vi "A170316-11_Auto.vi"() -> ()   [LabVIEW 2020]
uses:
  2e0b5f5e-2208-4490-a798-25a802626be8.vi
  Global_Variable/A170316-11.vi
  Global_Variable/Global.vi
  Database/Global1.vi
  <vilib>/addons/database/Connection.llb/DB Tools Open Connec (String).vi
  <vilib>/addons/database/NI_Database_API.lvlib
  <vilib>/regexp/Match Regular Expression.xnode
panel:
  out "设备状态":u16
  out "请拾取O型圈":bool
  out "请拾取弹簧":bool
  in  "控制器支架":T1(ring)
  in  "ECU步骤":T2(ring)
  in  "装配步骤":T3(ring)
  out "产品型号":string
  in  "更换产品":refnum<vi>
  in  "前序OK？_ECU":string
  in  "前序OK？":string
  in  "Process":string[](array[string])
  in  "Code":string[](array[string])
  in  "User":string[](array[string])
  in  "Result":string[](array[string])
  in  "Device":string[](array[string])
  out "请安装挡片":bool
  in  "STEP2":string
  in  "STEP1":string
  out "请取降噪块1":bool
  out "电机安装螺栓3扭矩确认":bool
  out "控制器支架螺栓5拧紧确认":bool
  out "安装扎带并取走工件":bool
  out "涂色标":bool
  out "按启动按钮拍照确认":bool
  out "电机安装螺栓2扭矩确认":bool
  out "电机安装螺栓1扭矩确认":bool
  out "请安装锁紧螺母":bool
  out "请取降噪垫片2":bool
  out "请取降噪垫片1":bool
  out "请取锁紧块":bool
  out "安装弹性垫圈弹簧并按启动拍照":bool
  out "请取降噪块2":bool
  out "控制器支架涂色标":bool
  out "控制器支架螺栓4拧紧确认":bool
  out "控制器支架螺栓3拧紧确认":bool
  out "控制器支架螺栓2拧紧确认":bool
  out "控制器支架螺栓1拧紧确认":bool
  out "请安装推力滚针轴承":bool
  in  "更换布局":string
  out "请拍照确认":bool
  out "安装支架扎带安装":bool
  out "请安装弹簧":bool
  out "控制器支架安装线卡扎带":bool
  out "磨合次数":i32
  in  "判定结果":bool[][](array[boolean])=[[TRUE]]
  in  "STEP3":string
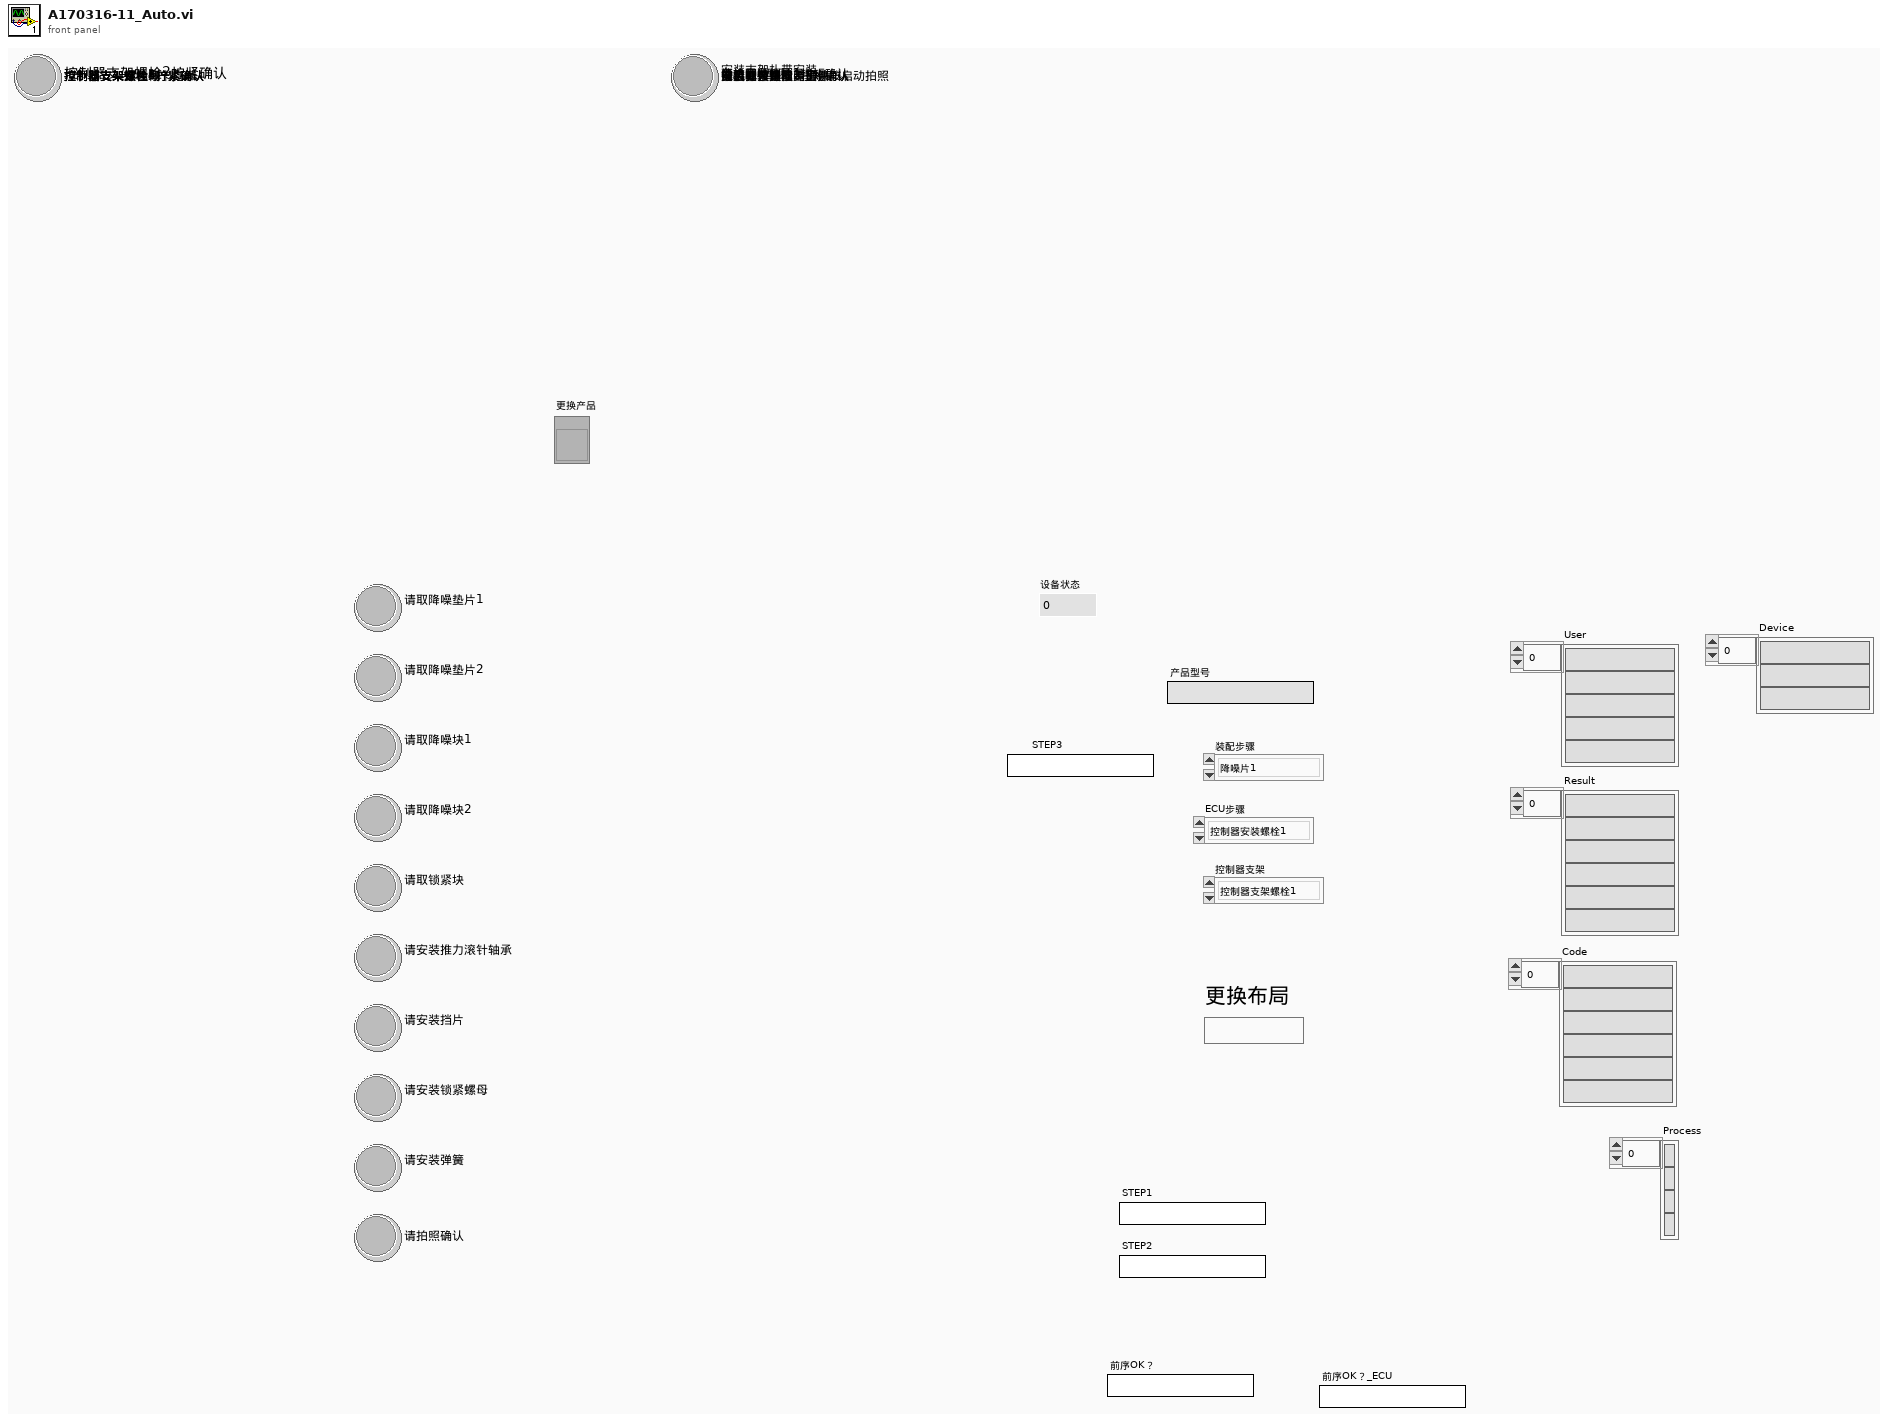
[diagram p1: front panel]
types:
  T1 = enum16{"控制器支架螺栓1", "控制器支架螺栓2", "控制器支架螺栓3", "控制器支架螺栓4", "控制器支架螺栓5", "涂色标", "安装线卡轧带", "完成"}
  T2 = enum16{"控制器安装螺栓1", "控制器安装螺栓2", "控制器安装螺栓3", "安装支架螺栓1", "安装支架螺栓2", "安装支架螺栓3", "安装支架螺栓4", "涂色标", "安装线卡轧带", "取走工件", "完成"}
  T3 = enum16{"降噪片1", "降噪片2", "降噪块1", "降噪块2", "锁紧块", "滚针轴承", "垫片", "锁紧螺母", "弹簧", "轴承拍照", "完成"}
  T4 = cluster{i64, i64, i64, "装配结果":string, "result string":string}
  T5 = cluster{i64, i64, i64, "装配结果":string, "result string":string}[]
  T6 = typedef "NI_Database_API.lvlib/Conn ObjectReference.ctl" = refnum<k1>
  T7 = cluster{i64, i64, i64, "ECU工位生产结果":string, "result string":string}
  T8 = cluster{i64, i64, i64, "ECU工位生产结果":string, "result string":string}[]
  T9 = cluster{"ECU工位生产结果":string, "result string":string}
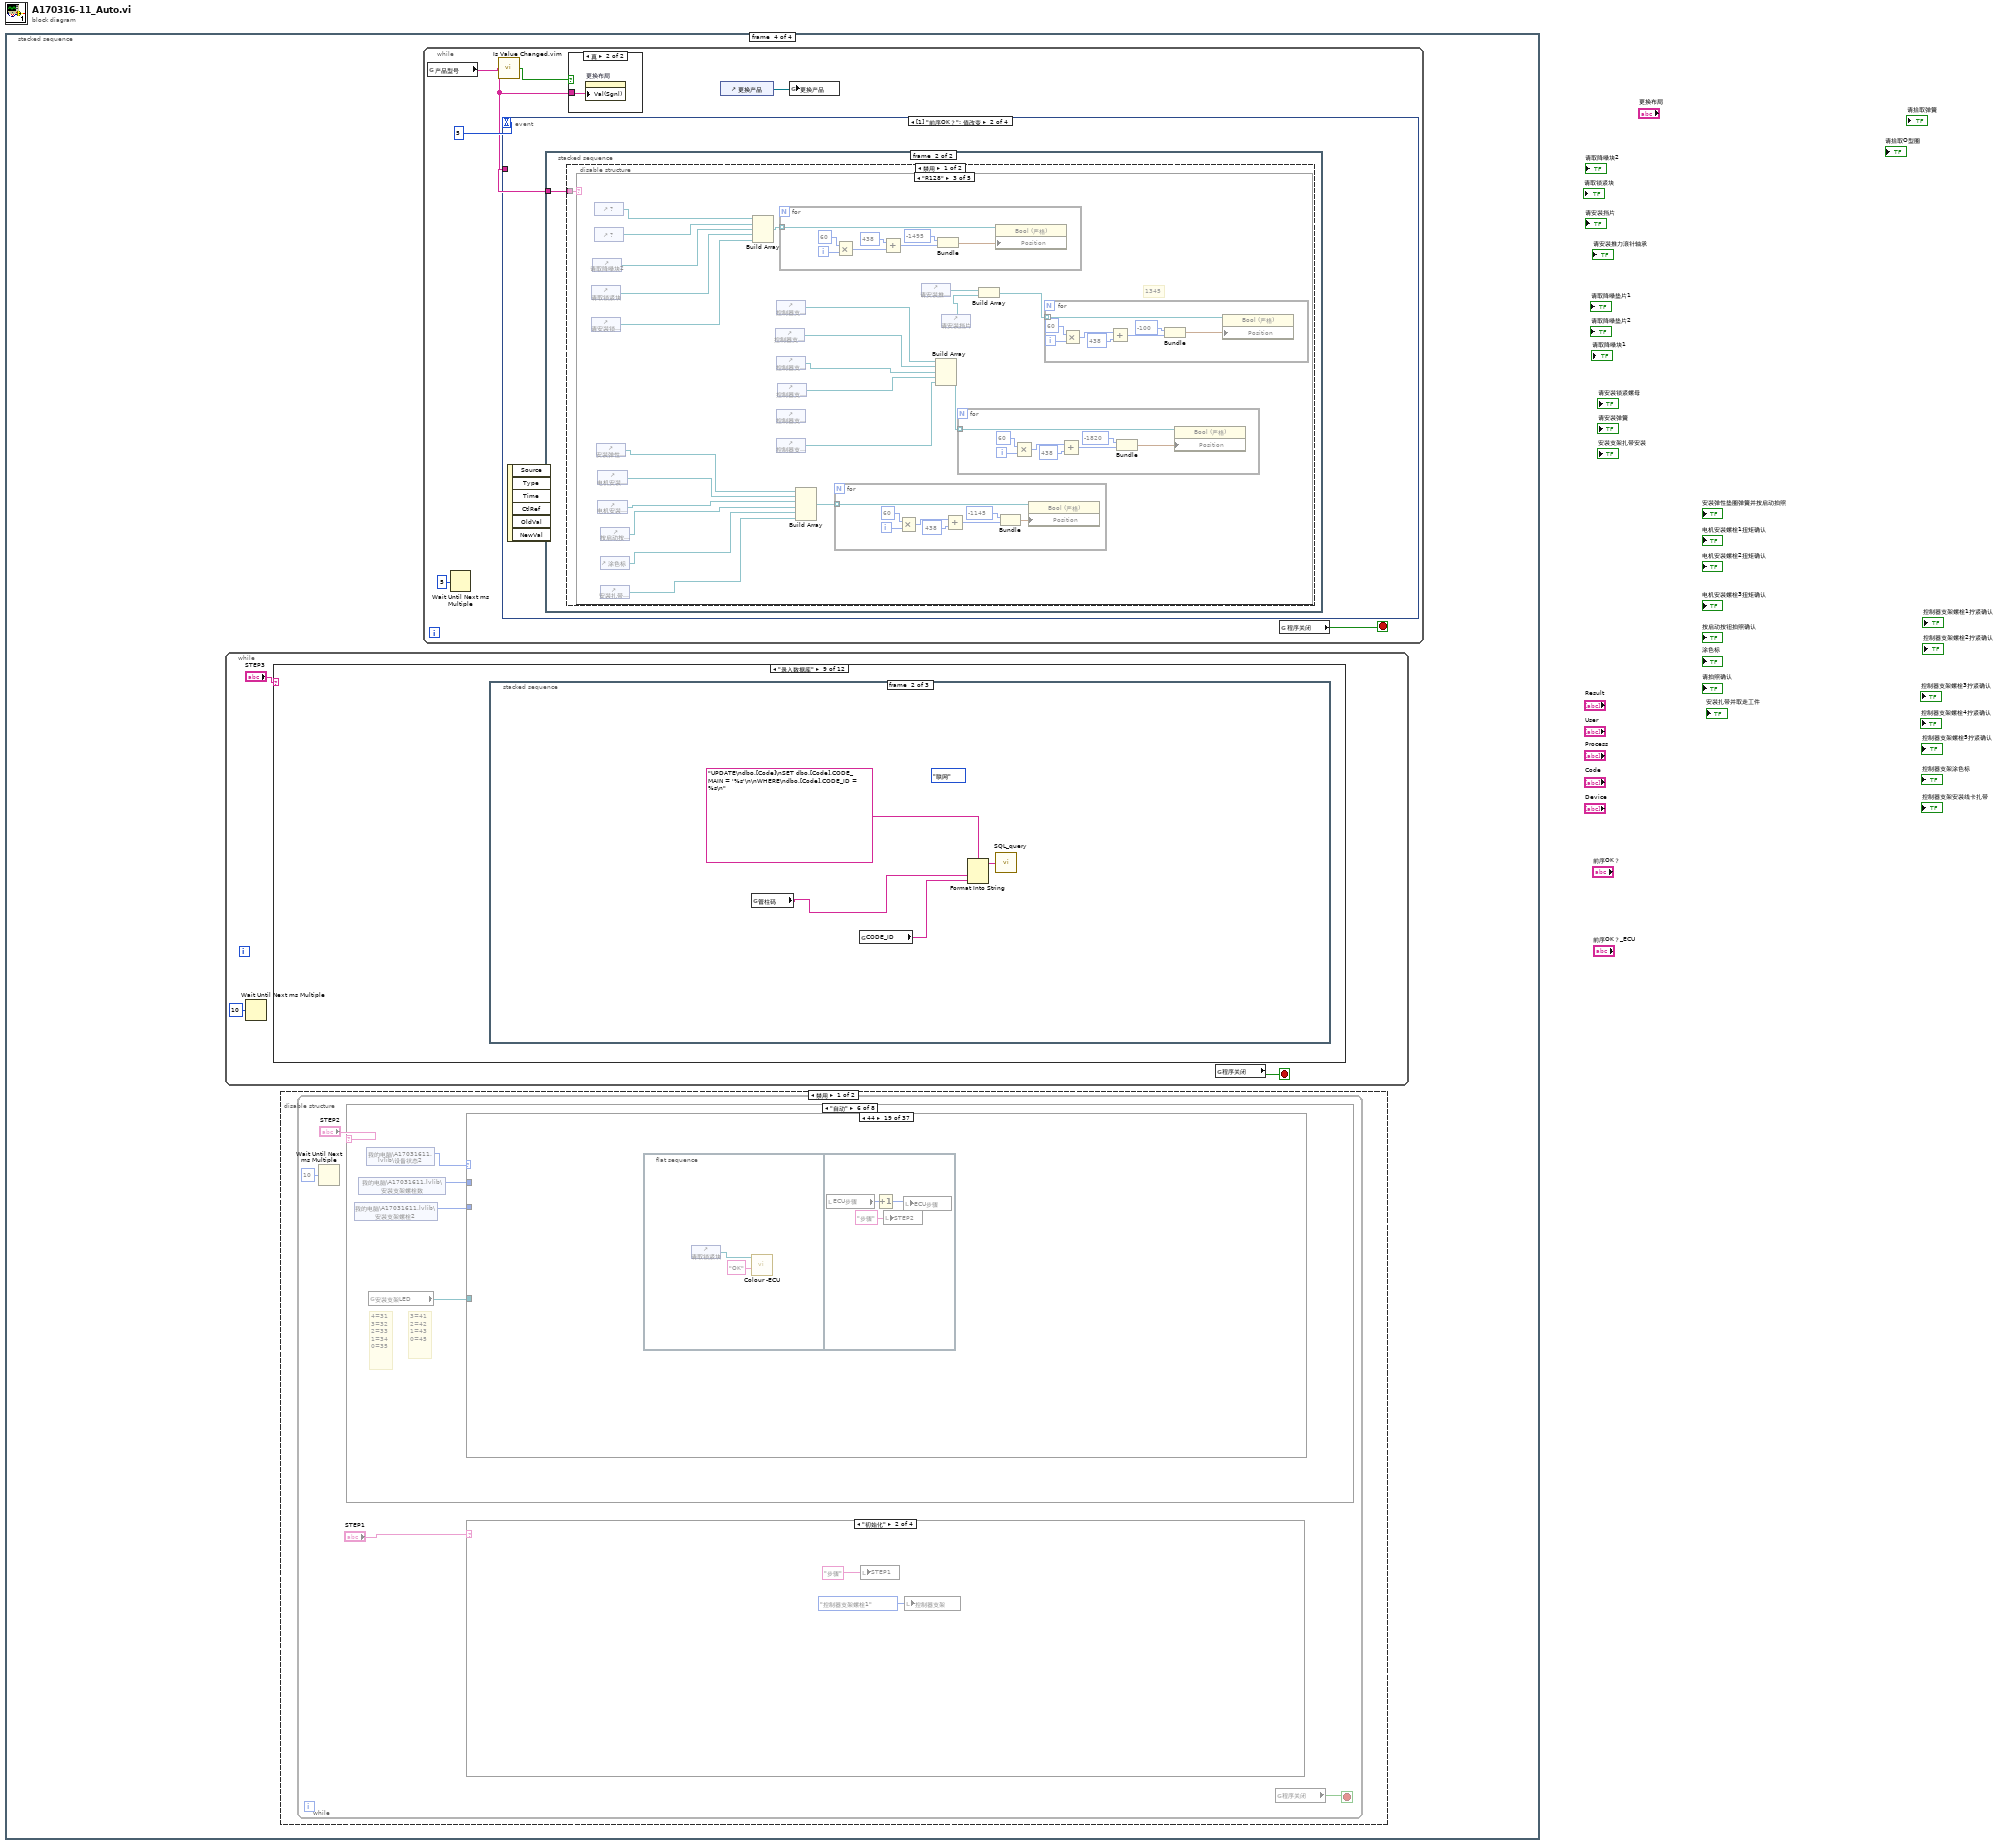
[diagram p0: block diagram]
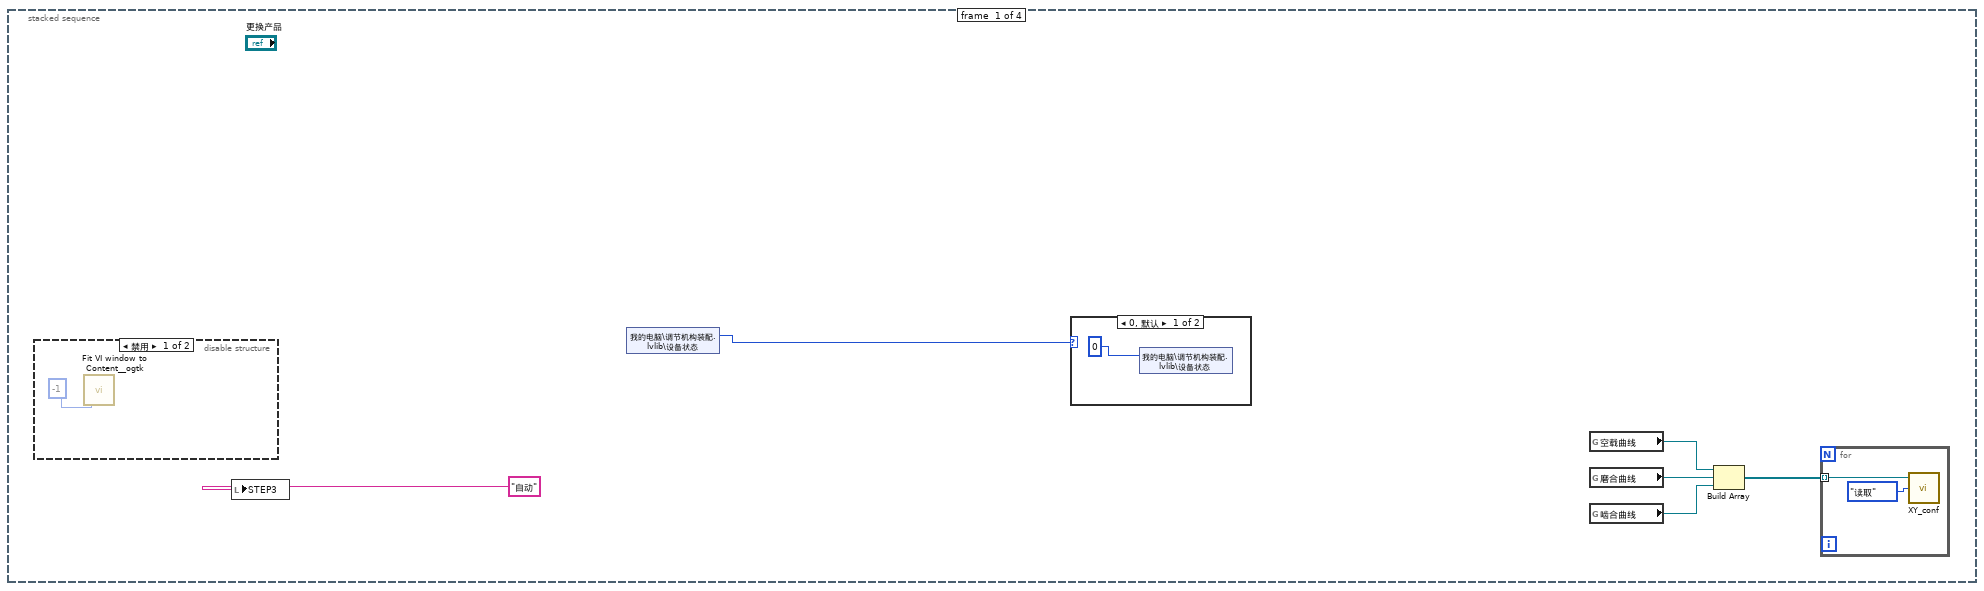
[diagram p2: hidden frame]
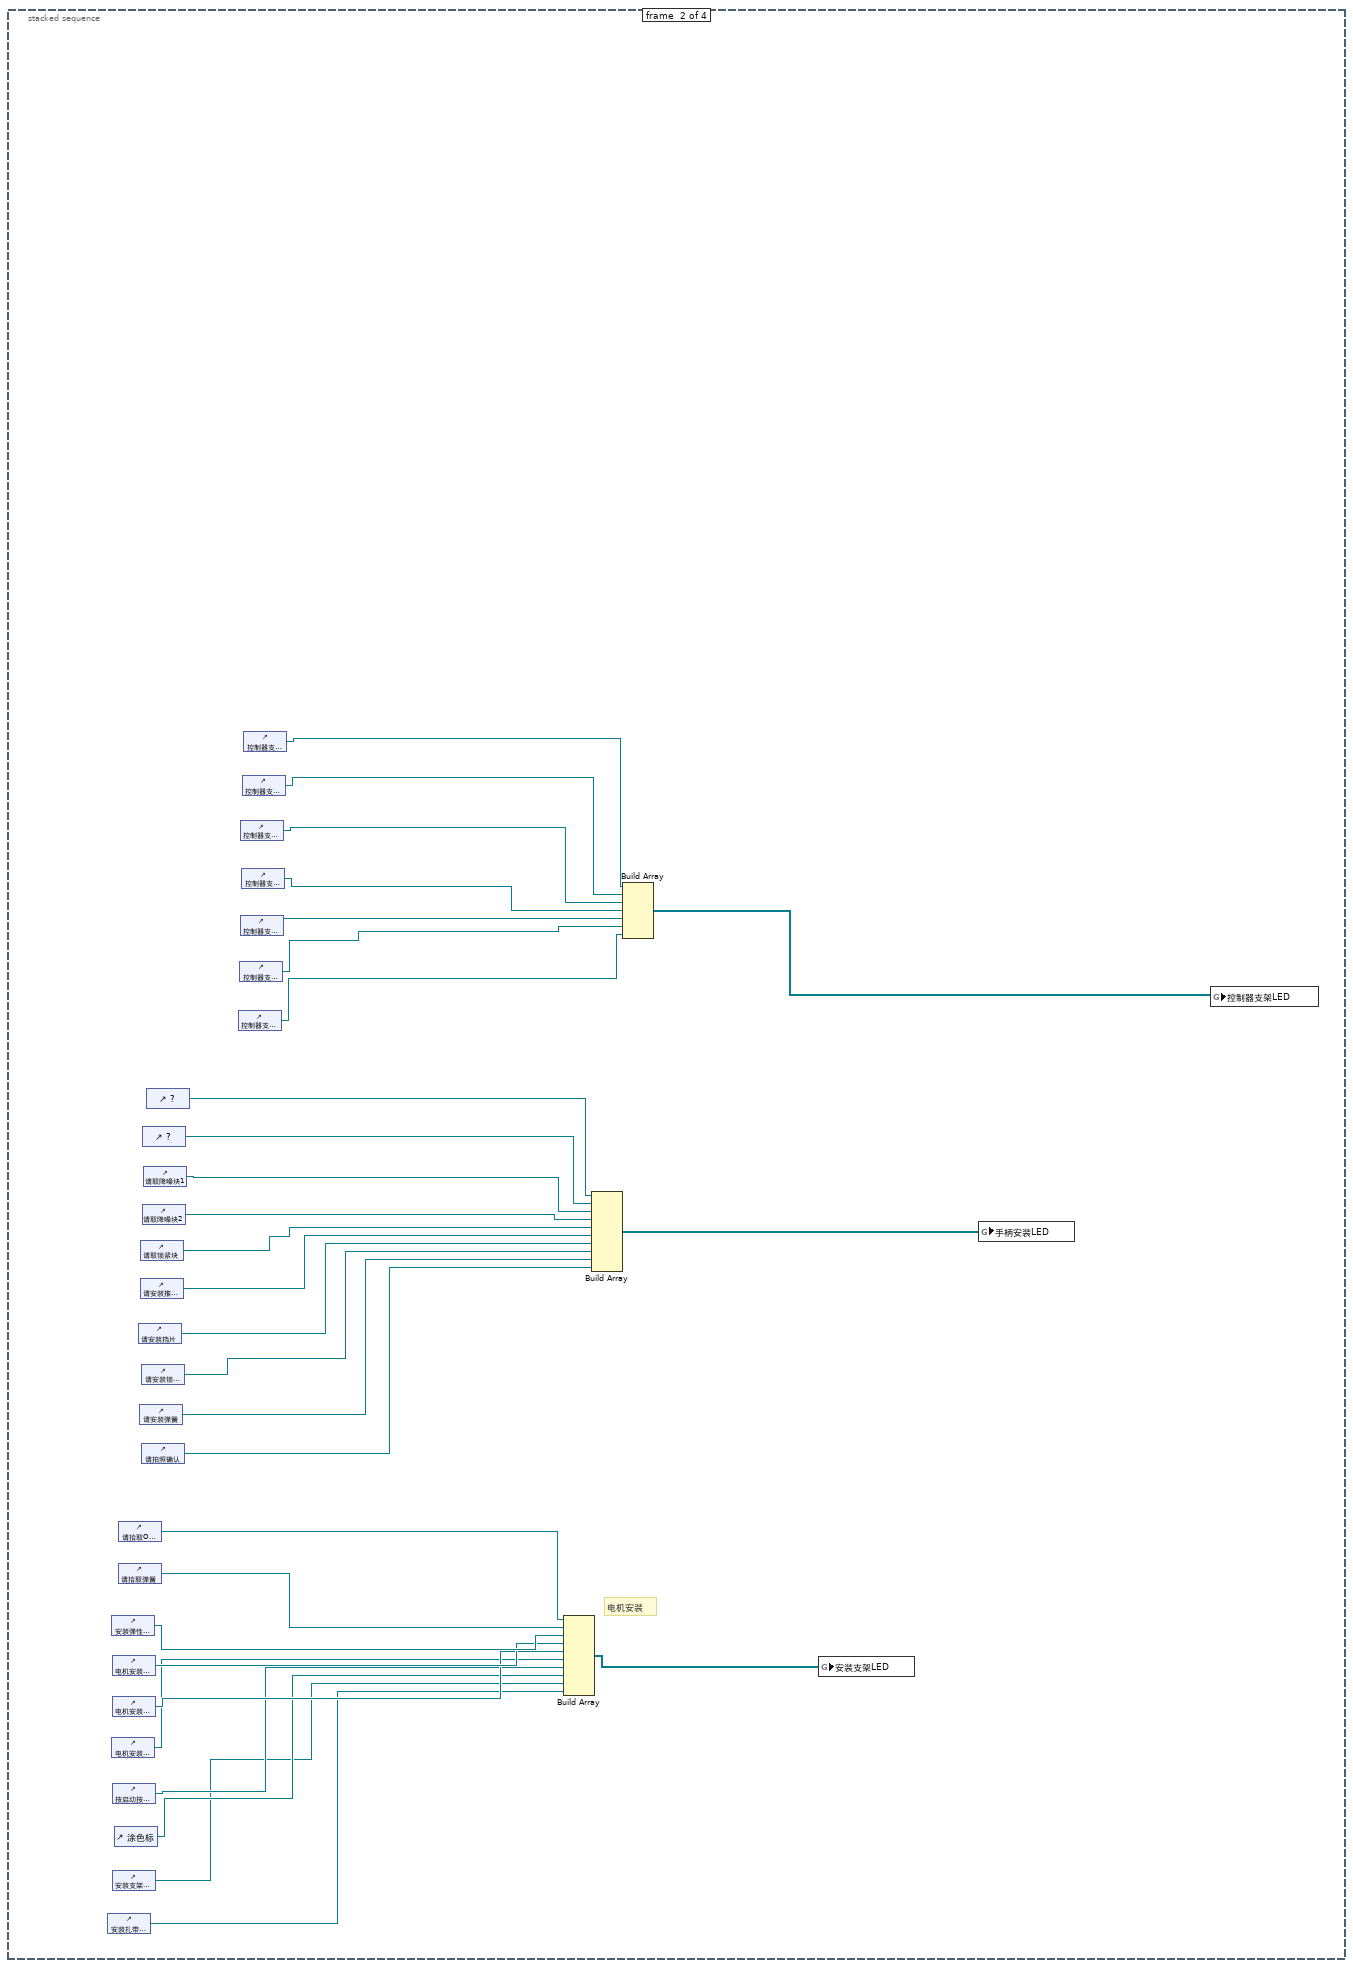
[diagram p5: hidden frame]
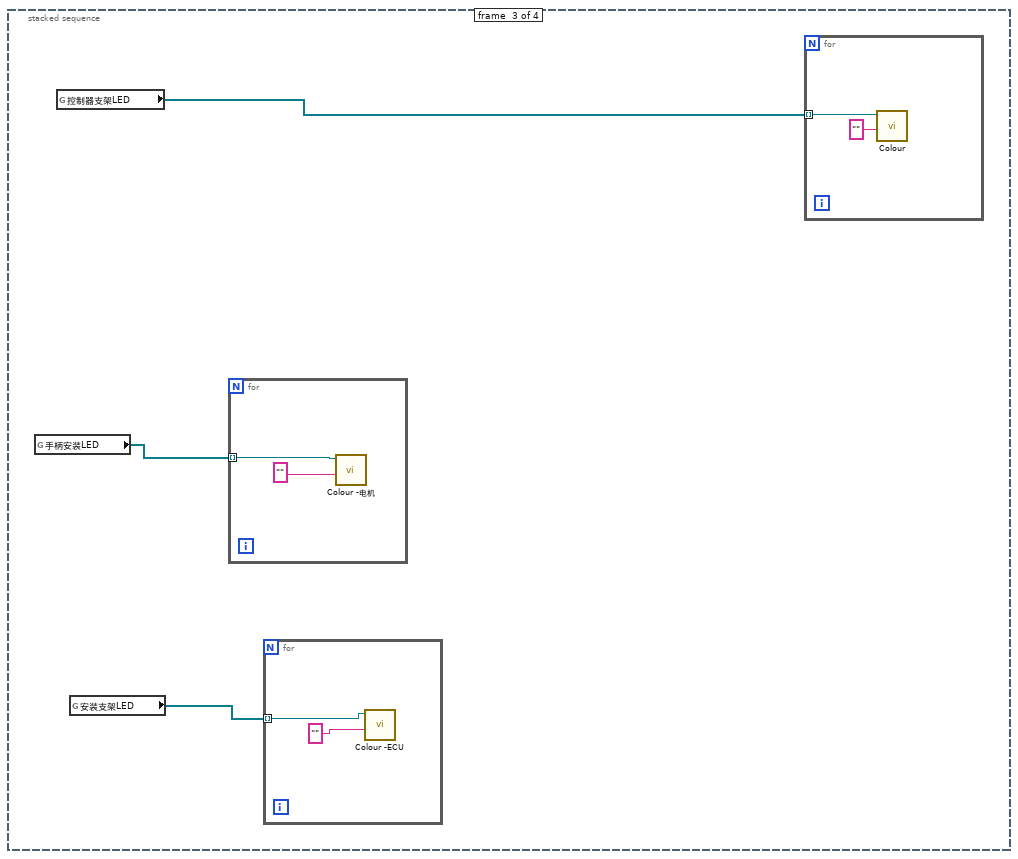
[diagram p6: hidden frame]
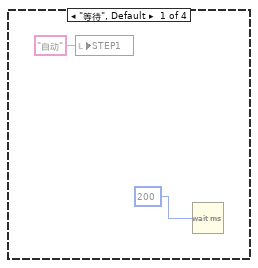
[diagram p7: hidden frame]
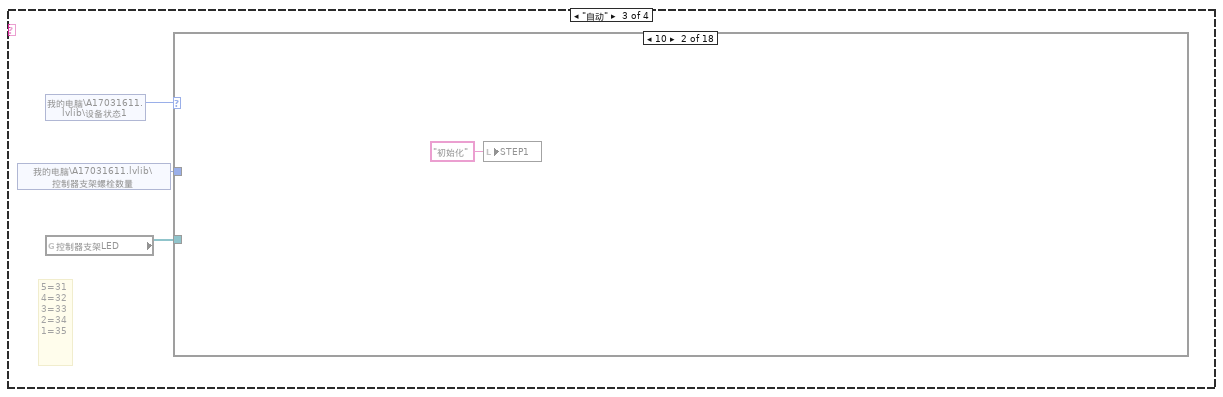
[diagram p8: hidden frame]
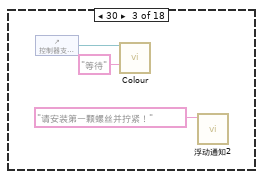
[diagram p10: hidden frame]
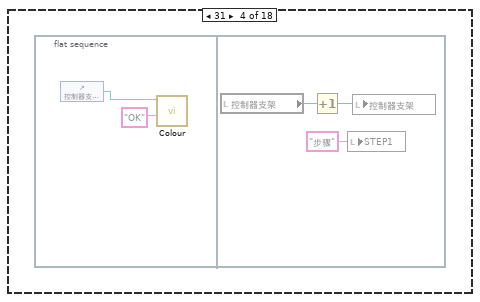
[diagram p11: hidden frame]
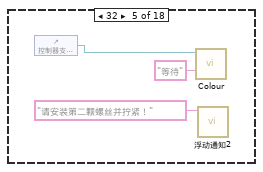
[diagram p12: hidden frame]
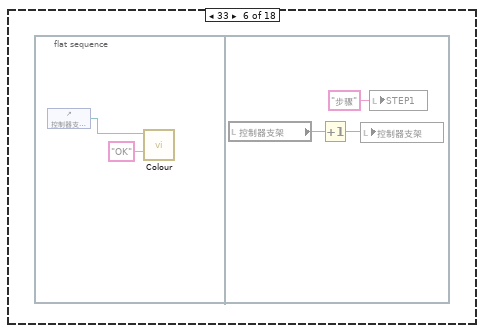
[diagram p13: hidden frame]
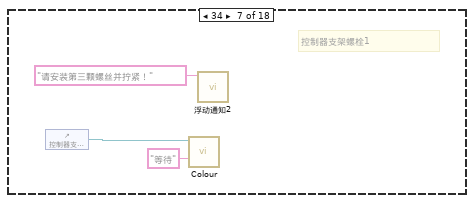
[diagram p14: hidden frame]
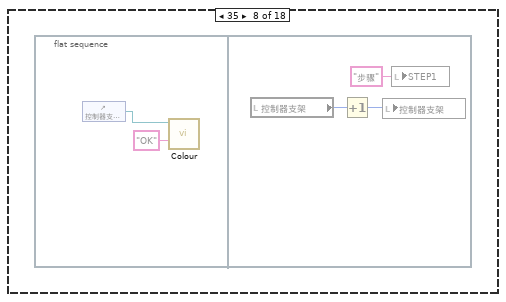
[diagram p15: hidden frame]
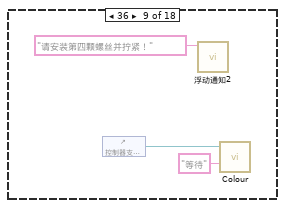
[diagram p16: hidden frame]
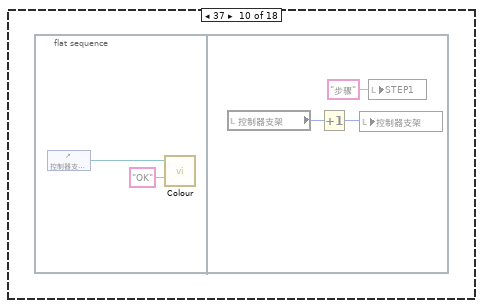
[diagram p17: hidden frame]
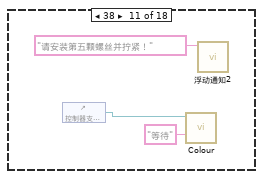
[diagram p18: hidden frame]
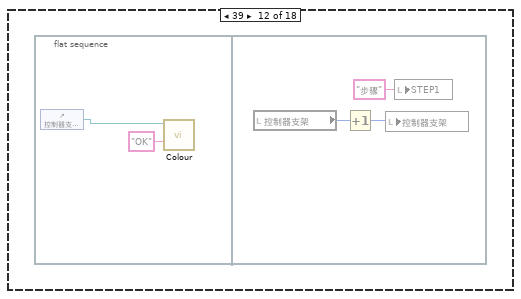
[diagram p19: hidden frame]
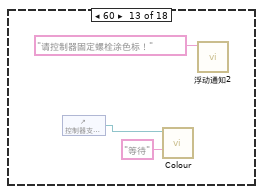
[diagram p20: hidden frame]
diagram:
  n1 = stacked-sequence {
    frame #0 {
      n2 = disable-structure shown="禁用" {
        frame Disabled {
          n3 = call "Fit VI window to Content__ogtk.vi"("border spacing (2 px)"=-1) -> ()  [unwired: 5 in, 2 out]
        }
        frame Enabled {
        }
      }
      n4 = local write "STEP3"("自动" ("STEP")) -> ()
      n5 = shared-variable "我的电脑\\调节机构装配.lvlib\\设备状态"() -> (w1:u16)  [unwired: 1 in, 1 out]
      n6 = case shown="0, 默认" w1 {
        frame 0, Default {
          n7 = shared-variable "我的电脑\\调节机构装配.lvlib\\设备状态"(i16 0 ("设备状态")) -> ()  [unwired: 1 in, 1 out]
        }
        frame 3721..3723 {
        }
      }
      n8 = global read "A170316-11.vi" "空载曲线"() -> (w2:refnum<vi>)
      n9 = global read "A170316-11.vi" "磨合曲线"() -> (w3:refnum<vi>)
      n10 = global read "A170316-11.vi" "啮合曲线"() -> (w4:refnum<vi>)
      n11 = Build Array(w2, w3, w4) -> (w5:refnum<vi>[])
      n12 = for {
        tunnel: w5 -> [w10] mode=indexing
        n13 = call "XY_conf.vi"("方式"=enum16{"写入", "读取"}."读取", "XY图引用"=w10) -> ()  [unwired: 3 in, 1 out]
      }
    }
    frame #1 {
      # "电机安装"
      n14 = control-ref of="安装扎带并取走工件"() -> (w25:refnum<vi>)
      n15 = control-ref of="安装弹性垫圈弹簧并按启动拍照"() -> (w32:refnum<vi>)
      n16 = control-ref of="电机安装螺栓3扭矩确认"() -> (w29:refnum<vi>)
      n17 = control-ref of="电机安装螺栓1扭矩确认"() -> (w31:refnum<vi>)
      n18 = control-ref of="电机安装螺栓2扭矩确认"() -> (w30:refnum<vi>)
      n19 = control-ref of="按启动按钮拍照确认"() -> (w28:refnum<vi>)
      n20 = control-ref of="安装支架扎带安装"() -> (w26:refnum<vi>)
      n21 = control-ref of="涂色标"() -> (w27:refnum<vi>)
      n22 = control-ref of="请拾取O型圈"() -> (w13:refnum<vi>)
      n23 = control-ref of="请拾取弹簧"() -> (w14:refnum<vi>)
      n24 = control-ref of="请安装挡片"() -> (w18:refnum<vi>)
      n25 = control-ref of="请安装弹簧"() -> (w16:refnum<vi>)
      n26 = control-ref of="请取锁紧块"() -> (w20:refnum<vi>)
      n27 = control-ref of="请安装推力滚针轴承"() -> (w19:refnum<vi>)
      n28 = control-ref of="请安装锁紧螺母"() -> (w17:refnum<vi>)
      n29 = control-ref of="请拍照确认"() -> (w15:refnum<vi>)
      n30 = control-ref of="?"() -> (w23:refnum<vi>)
      n31 = control-ref of="请取降噪块2"() -> (w21:refnum<vi>)
      n32 = control-ref of="请取降噪块1"() -> (w22:refnum<vi>)
      n33 = control-ref of="?"() -> (w24:refnum<vi>)
      n34 = control-ref of="控制器支架安装线卡扎带"() -> (w33:refnum<vi>)
      n35 = control-ref of="控制器支架涂色标"() -> (w34:refnum<vi>)
      n36 = control-ref of="控制器支架螺栓3拧紧确认"() -> (w37:refnum<vi>)
      n37 = control-ref of="控制器支架螺栓5拧紧确认"() -> (w35:refnum<vi>)
      n38 = control-ref of="控制器支架螺栓4拧紧确认"() -> (w36:refnum<vi>)
      n39 = control-ref of="控制器支架螺栓2拧紧确认"() -> (w38:refnum<vi>)
      n40 = control-ref of="控制器支架螺栓1拧紧确认"() -> (w39:refnum<vi>)
      n41 = Build Array(w13, w14, w32, w31, w30, w29, w28, w27, w26, w25) -> (w11:refnum<vi>[])
      n42 = Build Array(w24, w23, w22, w21, w20, w19, w18, w17, w16, w15) -> (w12:refnum<vi>[])
      n43 = Build Array(w39, w38, w37, w36, w35, w34, w33) -> (w40:refnum<vi>[])
      n44 = global write "A170316-11.vi" "安装支架LED"(w11) -> ()
      n45 = global write "A170316-11.vi" "手柄安装LED"(w12) -> ()
      n46 = global write "A170316-11.vi" "控制器支架LED"(w40) -> ()
    }
    frame #2 {
      n47 = global read "A170316-11.vi" "手柄安装LED"() -> (w42:refnum<vi>[])
      n48 = global read "A170316-11.vi" "控制器支架LED"() -> (w43:refnum<vi>[])
      n49 = global read "A170316-11.vi" "安装支架LED"() -> (w41:refnum<vi>[])
      n50 = for {
        tunnel: w42 -> [w47] mode=indexing
        n51 = call "Colour -电机.vi"("result"="", "colourRef"=w47) -> ()  [unwired: 9 in, 1 out]
      }
      n52 = for {
        tunnel: w41 -> [w45] mode=indexing
        n53 = call "Colour -ECU.vi"("result"="", "colourRef"=w45) -> ()  [unwired: 9 in, 1 out]
      }
      n54 = for {
        tunnel: w43 -> [w48] mode=indexing
        n55 = call "Colour.vi"("result"="", "colourRef"=w48) -> ()  [unwired: 9 in, 1 out]
      }
    }
    frame #3 {
      n56 = while {
        stop <- w633 stop-if-true
        n57 = Wait Until Next ms Multiple(millisecond multiple=u32 10 ("毫秒倍数")) -> ()  [unwired: 1 out]
        n58 = case shown="\"录入数据库\"" "STEP3" {
          frame "等待", Default {
            n59 = local write "STEP3"("自动" ("STEP")) -> ()
            n60 = Wait (ms)(milliseconds to wait=u32 200 ("等待时间（毫秒）")) -> ()  [unwired: 1 out]
          }
          frame "手动" {
            n61 = global read "Global.vi" "ECU自动"() -> (w640:refnum<vi>)
            n62 = property class="Bool (严格)"(reference=w640, "Value"=FALSE) -> ()  [unwired: 1 in, 2 out]
            n63 = local write "STEP1"("等待" ("STEP1")) -> ()
            n64 = shared-variable "我的电脑\\调节机构装配.lvlib\\设备状态"(u16 0 ("设备状态")) -> ()  [unwired: 1 in, 1 out]
            n65 = global read "Global.vi" "电机程序自动"() -> (w642:refnum<vi>)
            n66 = property class="Bool"(reference=w642, "Value"=FALSE) -> ()  [unwired: 1 in, 2 out]
            n67 = local write "STEP3"("等待" ("STEP")) -> ()
            n68 = Wait (ms)(milliseconds to wait=u32 100 ("等待时间（毫秒）")) -> ()  [unwired: 1 out]
          }
          frame "初始化" {
            n69 = stacked-sequence {
              frame #0 {
                w655 = enum16{"录入", "清空"}."清空" ("功能")
                n70 = global read "Global.vi" "装配前序显示字"() -> (w646:refnum<vi>)
                n71 = shared-variable "我的电脑\\Global.lvlib\\工位追溯码"("" ("传感器码")) -> ()  [unwired: 1 in, 1 out]
                n72 = call "物料信息录入.vi"("功能"=w655) -> ("错误输出"=w654:errorcluster)  [unwired: 14 in]
                n73 = call "质量信息录入.vi"("功能"=w655, "错误输入（无错误）"=w654) -> ("错误输出"=w656:errorcluster)  [unwired: 13 in]
                n74 = property class="Str"(reference=w646, "Value"="" ("值")) -> (reference out=w645:refnum<vi>)  [unwired: 1 in, 1 out]
                n75 = call "不合格信息录入.vi"("功能"=w655, "错误输入（无错误）"=w656) -> ()  [unwired: 13 in, 1 out]
                n76 = property class="Str"(reference=w645, "Text.BGColor"=u32 16777216 ("文本.文本颜色:背景色")) -> ()  [unwired: 1 in, 2 out]
                n77 = global read "Global.vi" "电机程序自动"() -> (w652:refnum<vi>)
                n78 = global read "Global.vi" "检测结果"() -> (w650:refnum<vi>)
                n79 = property class="Bool"(reference=w652, "Value"=TRUE) -> ()  [unwired: 1 in, 2 out]
                n80 = call "Colour.vi"("result"="", "colourRef"=w650) -> ()  [unwired: 9 in, 1 out]
              }
              frame #1 {
                n81 = global read "A170316-11.vi" "手柄安装LED"() -> (w657:refnum<vi>[])
                n82 = for {
                  tunnel: w657 -> [w659] mode=indexing
                  n83 = call "Colour -电机.vi"("result"="", "colourRef"=w659) -> ()  [unwired: 9 in, 1 out]
                }
              }
              frame #2 {
                n84 = global read "Global.vi" "Result"() -> (w663:refnum<vi>)
                n85 = property class="Tbl"(reference=w663, "Value"=string[][] []) -> (reference out=w664:refnum<vi>, error out=w665:errorcluster)  [unwired: 1 in]
                n86 = property class="Tbl"(reference=w664, error in=w665, "Row Headers[]"=string[] ["正向空载扭矩最大值", "正向空载扭矩最小值", "正向空载扭矩平均值", "正向空载扭矩波动值", "逆向空载扭矩最大值", "逆向空载扭矩最小值", "逆向空载扭矩平均值", "逆向空载扭矩波动值", "啮合间隙"] ("列首字符串[]")) -> ()  [unwired: 2 out]
                n87 = local write "装配步骤"(T3."降噪片1" ("装配步骤")) -> ()
              }
              frame #3 {
                n88 = local write "STEP3"("等待" ("STEP")) -> ()
              }
            }
          }
          frame "批次数量判断" {
            n89 = shared-variable "我的电脑\\Global.lvlib\\产品型号"() -> (w672:string, error out=w675:errorcluster)  [unwired: 1 in]
            n90 = global read "Global.vi" "批次"() -> (w673:refnum<vi>)
            n91 = call "获取批次信息.vi"("error in (no error)"=w675, "产品型号"=w672, "Tbl引用句柄"=w673) -> ("error out"=w674:errorcluster)  [unwired: 7 in, 1 out]
            n92 = property class="Tbl"(reference=w673, error in=w674) -> ("Value"=w676:string[][])  [unwired: 2 out]
            n93 = for {
              tunnel: w676 -> [w682] mode=indexing
              tunnel: [w677] -> w671 mode=indexing
              n94 = Index Array(array=w682) -> (element #1=w678:string, element #3=w681:string)  [unwired: 3 in, 1 out]
              n95 = Decimal String To Number(string=w681) -> (number=w680:i32)  [unwired: 2 in, 1 out]
              n96 = Less Or Equal To 0?(x=w680) -> (x <= 0?=w679:bool)
              n97 = case shown="真" w679 {
                tunnel: w678 -> [_ w687]
                tunnel: [TRUE FALSE] -> w677
                frame False {
                }
                frame True {
                  n98 = Concatenate Strings(w687, "数量不足！" ("字符串")) -> (w685:string)
                  n99 = One Button Dialog(message=w685) -> ()  [unwired: 1 in, 1 out]
                }
              }
            }
            n100 = And Array Elements(Boolean array=w671) -> (logical AND=w670:bool)
            n101 = Select(t="扫码" ("STEP"), s=w670, f="手动" ("STEP")) -> (s? t:f=w667:string)
            n102 = local write "STEP3"(w667) -> ()
          }
          frame "扫管柱码" {
            n103 = stacked-sequence {
              frame #0 {
                w690 = "请扫管柱码！" ("提示信息")
                n104 = global read "Global.vi" "管柱码"() -> (w689:refnum<vi>)
                n105 = global read "Global1.vi" "联机模式"() -> (w691:enum16{"单机", "追溯"})
                n106 = call "输入框.vi"("提示信息"=w690) -> ("条形码输出"=w688:string)
                n107 = property class="Str"(reference=w689, "Text.Text"=w688) -> ()  [unwired: 1 in, 2 out]
                n108 = shared-variable "我的电脑\\Global.lvlib\\工位追溯码"(w688) -> ()  [unwired: 1 in, 1 out]
                n109 = global write "Global1.vi" "管柱码"(w688) -> ()
                n110 = call "浮动通知.vi"("通知内容"=w690) -> ()  [unwired: 11 in]
                n111 = case shown="\"\", 默认" w688 {
                  selector: w688 -> [w695 _]
                  tunnel: [w694 "手动"] -> w692
                  tunnel: w691 -> [w693 _]
                  frame "", Default {
                    n112 = Wait (ms)(milliseconds to wait=u32 50 ("等待时间（毫秒）")) -> ()  [unwired: 1 out]
                    n113 = case shown="\"追溯\"" w693 {
                      tunnel: w695 -> [_ w702]
                      tunnel: ["步骤" ("State(s) in Front (\"\")") w701] -> w694
                      frame "单机", Default {
                      }
                      frame "追溯" {
                        n114 = global read "Global1.vi" "前序DEVICE_ID"() -> (w700:string)
                        n115 = Equal?(x=w700, y="") -> (x = y?=w698:bool)
                        n116 = case shown="真" w698 {
                          tunnel: w702 -> [w704 w746]
                          tunnel: [w703 w745] -> w701
                          frame False {
                            n117 = stacked-sequence {
                              tunnel: w704 -> [w712 _ _]
                              tunnel: [_ _ w725] -> w703
                              frame #0 {
                                n118 = global read "Global1.vi" "PRODUCT_ID"() -> (w709:string)
                                n119 = Format Into String(format string="SELECT\ndbo.[Code].CODE_ID\nFROM\ndbo.[Code]\nWHERE\ndbo.[Code].CODE_MAIN = '%s'\nAND\ndbo.[Code].PRODUCT_ID = %s\n" ("格式字符串"), w712, w709) -> (resulting string=w711:string)  [unwired: 2 in, 1 out]
                                n120 = call "SQL_query.vi"("SQL query"=w711, "联机模式"=enum16{"单机", "追溯"}."追溯") -> ("data"=w714:string[][])  [unwired: 1 in, 2 out]
                                n121 = Index Array(array=w714, index (row)=0 ("索引 (行)")) -> (element=w713:string[])  [unwired: 1 in]
                                n122 = Index Array(array=w713, index=0 ("索引")) -> (element=w706:string)
                                n123 = global write "Global1.vi" "CODE_ID"(w706) -> ()
                              }
                              frame #1 {
                                (unwired) enum16{"单机", "联网"}."联网" ("联机模式")
                                n124 = global read "Global1.vi" "前序DEVICE_ID"() -> (w715:string)
                                n125 = global read "Global1.vi" "CODE_ID"() -> (w716:string)
                                n126 = Format Into String(format string="SELECT\ndbo.[Result].RESULT_VALUE\nFROM\ndbo.[Result]\nWHERE\ndbo.[Result].DEVICE_ID = '%s'\nAND\ndbo.[Result].CODE_ID = %s\n" ("格式字符串"), w715, w716) -> (resulting string=w721:string)  [unwired: 2 in, 1 out]
                                n127 = call "SQL_query.vi"("SQL query"=w721) -> ("data"=w723:string[][])  [unwired: 2 in, 2 out]
                                n128 = Index Array(array=w723, index (row)=0 ("索引 (行)")) -> (element=w722:string[])  [unwired: 1 in]
                                n129 = Index Array(array=w722, index=0 ("索引")) -> (element=w717:string)
                                n130 = local write "前序OK？"(w717) -> ()
                              }
                              frame #2 {
                                n131 = local read "前序OK？"() -> (w724:string)
                                n132 = case shown="\"OK\"" w724 {
                                tunnel: ["等待" "等待" "步骤"] -> w725
                                frame Default {
                                n133 = global read "Global.vi" "装配前序显示字"() -> (w729:refnum<vi>)
                                n134 = property class="Str"(reference=w729, "Value"="漏序 " ("值")) -> (reference out=w727:refnum<vi>)  [unwired: 1 in, 1 out]
                                n135 = Wait (ms)(milliseconds to wait=u32 2000 ("等待时间（毫秒）")) -> ()  [unwired: 1 out]
                                n136 = call "浮动通知.vi"("通知内容"="上序漏序！！" ("Status")) -> ()  [unwired: 11 in]
                                n137 = property class="Str"(reference=w727, "Text.BGColor"=u32 16772608 ("文本.文本颜色:背景色")) -> ()  [unwired: 1 in, 2 out]
                                }
                                frame "NG" {
                                (unwired) i16 6 ("设备状态控制字")
                                n138 = global read "Global.vi" "装配前序显示字"() -> (w736:refnum<vi>)
                                n139 = property class="Str"(reference=w736, "Value"="不合格 " ("值")) -> (reference out=w734:refnum<vi>)  [unwired: 1 in, 1 out]
                                n140 = call "浮动通知.vi"("通知内容"="上序生产结果不合格！" ("Status")) -> ()  [unwired: 11 in]
                                n141 = property class="Str"(reference=w734, "Text.BGColor"=u32 16711680 ("文本.文本颜色:背景色")) -> ()  [unwired: 1 in, 2 out]
                                n142 = Wait (ms)(milliseconds to wait=u32 2000 ("等待时间（毫秒）")) -> ()  [unwired: 1 out]
                                }
                                frame "OK" {
                                n143 = global read "Global.vi" "装配前序显示字"() -> (w743:refnum<vi>)
                                n144 = property class="Str"(reference=w743, "Value"="合格" ("值")) -> (reference out=w741:refnum<vi>)  [unwired: 1 in, 1 out]
                                n145 = property class="Str"(reference=w741, "Text.BGColor"=u32 6618880 ("文本.文本颜色:背景色")) -> ()  [unwired: 1 in, 2 out]
                                }
                                }
                              }
                            }
                          }
                          frame True {
                            n146 = stacked-sequence {
                              tunnel: w746 -> [w748 w749 _]
                              tunnel: [_ _ "步骤"] -> w745
                              frame #0 {
                                n147 = global read "Global1.vi" "PRODUCT_ID"() -> (w747:string)
                                n148 = call "INTOCODE.vi"("CODE_MAIN"=w748, "PRODUCT_ID"=w747) -> ()  [unwired: 13 in, 1 out]
                              }
                              frame #1 {
                                n149 = global read "Global1.vi" "PRODUCT_ID"() -> (w755:string)
                                n150 = Format Into String(format string="SELECT\ndbo.[Code].CODE_ID\nFROM\ndbo.[Code]\nWHERE\ndbo.[Code].CODE_MAIN = '%s'\nAND\ndbo.[Code].PRODUCT_ID = %s\n" ("格式字符串"), w749, w755) -> (resulting string=w756:string)  [unwired: 2 in, 1 out]
                                n151 = call "SQL_query.vi"("SQL query"=w756, "联机模式"=enum16{"单机", "追溯"}."追溯") -> ("data"=w758:string[][])  [unwired: 1 in, 2 out]
                                n152 = Index Array(array=w758, index (row)=0 ("索引 (行)")) -> (element=w757:string[])  [unwired: 1 in]
                                n153 = Index Array(array=w757, index=0 ("索引")) -> (element=w754:string)
                                n154 = global write "Global1.vi" "CODE_ID"(w754) -> ()
                              }
                              frame #2 {
                                (unwired) "请扫管柱码！" ("提示信息")
                                n155 = global read "Global.vi" "装配前序显示字"() -> (w763:refnum<vi>)
                                n156 = property class="Str"(reference=w763, "Value"="首序" ("值")) -> (reference out=w761:refnum<vi>)  [unwired: 1 in, 1 out]
                                n157 = property class="Str"(reference=w761, "Text.BGColor"=u32 6618880 ("文本.文本颜色:背景色")) -> ()  [unwired: 1 in, 2 out]
                              }
                            }
                          }
                        }
                      }
                    }
                  }
                  frame "exit" {
                  }
                }
                n158 = local write "STEP3"(w692) -> ()
              }
              frame #1 {
                n159 = Wait (ms)(milliseconds to wait=u32 100 ("等待时间（毫秒）")) -> ()  [unwired: 1 out]
              }
            }
          }
          frame "扫电机码" {
            n160 = stacked-sequence {
              frame #0 {
                w766 = "请扫电机码！" ("提示信息")
                n161 = call "输入框.vi"("提示信息"=w766) -> ("条形码输出"=w767:string)
                n162 = call "浮动通知.vi"("通知内容"=w766) -> ()  [unwired: 11 in]
                n163 = case shown="\"\", 默认" w767 {
                  selector: w767 -> [w769 _]
                  tunnel: [w770 "手动"] -> w768
                  frame "", Default {
                    n164 = global read "Global1.vi" "联机模式"() -> (w771:enum16{"单机", "追溯"})
                    n165 = shared-variable "我的电脑\\Global.lvlib\\电机码"(w769) -> ()  [unwired: 1 in, 1 out]
                    n166 = global write "Global1.vi" "电机码"(w769) -> ()
                    n167 = case shown="\"单机\", 默认" w771 {
                      tunnel: w769 -> [_ _]
                      tunnel: ["等待" ("State(s) in Front (\"\")") "等待" ("State(s) in Front (\"\")")] -> w770
                      frame "单机", Default {
                      }
                      frame "追溯" {
                        n168 = disable-structure shown="禁用" {
                          frame Disabled {
                            n169 = shared-variable "我的电脑\\A17031611.lvlib\\电机安装螺栓数量"() -> (w774:i16)  [unwired: 1 in, 1 out]
                            n170 = case shown="2, 默认" w774 {
                              frame 2, Default {
                                n171 = shared-variable "我的电脑\\A17031611.lvlib\\设备状态3"(i16 41 ("设备状态控制字")) -> ()  [unwired: 1 in, 1 out]
                              }
                              frame 3 {
                                n172 = shared-variable "我的电脑\\A17031611.lvlib\\设备状态3"(i16 40 ("设备状态控制字")) -> ()  [unwired: 1 in, 1 out]
                              }
                            }
                          }
                          frame Enabled {
                          }
                        }
                      }
                    }
                  }
                  frame "exit" {
                  }
                }
                n173 = local write "STEP3"(w768) -> ()
              }
              frame #1 {
                n174 = Wait (ms)(milliseconds to wait=u32 100 ("等待时间（毫秒）")) -> ()  [unwired: 1 out]
              }
            }
          }
          frame "录入批次" {
            n175 = shared-variable "我的电脑\\Global.lvlib\\产品型号"() -> (w780:string)  [unwired: 1 in, 1 out]
            n176 = call "更新批次.vi"("型号"=w780) -> ("error out"=w781:errorcluster)  [unwired: 10 in]
            n177 = call "更新易损件.vi"("error in (no error)"=w781) -> ("error out"=w784:errorcluster)  [unwired: 10 in]
            n178 = global read "Global.vi" "批次"() -> (w782:refnum<vi>)
            n179 = property class="Tbl"(reference=w782, error in=w784) -> ("Value"=w783:string[][])  [unwired: 2 out]
            n180 = for {
              tunnel: w783 -> [w787] mode=indexing
              n181 = Index Array(array=w787) -> (element #1=w786:string, element #2=w785:string)  [unwired: 2 in]
              n182 = call "物料信息录入.vi"("物料名称"=w786, "功能"=enum16{"录入", "清空"}."录入", "物料编码"=w785) -> ()  [unwired: 12 in, 1 out]
            }
            n183 = local write "STEP3"("等待" ("STEP")) -> ()
          }
          frame "自动" {
            n184 = shared-variable "我的电脑\\调节机构装配.lvlib\\设备状态"() -> (w789:u16)  [unwired: 1 in, 1 out]
            "设备状态" <- w789
            n185 = global read "A170316-11.vi" "手柄安装LED"() -> (w790:refnum<vi>[])
            n186 = case shown="200" w789 {
              tunnel: w790 -> [_ _ _ _ w795 w804 w808 w819 _ _ _ _ _ _ _ _ _ _ _ _ _ _ _ _ _ _ w878 _ _ _ _ _ _ _ w913 w919 _ _ w931 _ w941 w944 _ _ _ w974 _ _ _ _ _]
              frame 0 {
              }
              frame 5 {
                n187 = local write "STEP3"("初始化" ("STEP3")) -> ()
              }
              frame 4 {
                n188 = call "浮动通知.vi"("通知内容"="复位完成" ("Status")) -> ()  [unwired: 11 in]
              }
              frame 6 {
                n189 = local write "STEP3"("扫管柱码" ("STEP3")) -> ()
              }
              frame 7 {
                n190 = global read "Global.vi" "产品型号"() -> (w796:string)
                n191 = Index Array(array=w795) -> (element=w794:refnum<vi>)  [unwired: 1 in]
                n192 = case shown="\"R567X\", 默认" w796 {
                  tunnel: w794 -> [w797 w800]
                  frame "R567X", Default {
                    n193 = call "浮动通知.vi"("通知内容"="请取降噪垫片1") -> ()  [unwired: 11 in]
                    n194 = call "Colour -电机.vi"("result"="等待", "colourRef"=w797) -> ()  [unwired: 9 in, 1 out]
                  }
                  frame "R563X" {
                    n195 = call "浮动通知.vi"("通知内容"="请取衬套1") -> ()  [unwired: 11 in]
                    n196 = call "Colour -电机.vi"("result"="等待", "colourRef"=w800) -> ()  [unwired: 9 in, 1 out]
                  }
                }
              }
              frame 8 {
                n197 = Index Array(array=w804) -> (element=w803:refnum<vi>)  [unwired: 1 in]
                n198 = call "Colour -电机.vi"("result"="OK", "colourRef"=w803) -> ()  [unwired: 9 in, 1 out]
              }
              frame 9 {
                n199 = global read "Global.vi" "产品型号"() -> (w809:string)
                n200 = Index Array(array=w808, index=1 ("索引")) -> (element=w806:refnum<vi>)
                n201 = case shown="\"R563X\"" w809 {
                  tunnel: w806 -> [w810 w813]
                  frame "R567X", Default {
                    n202 = call "浮动通知.vi"("通知内容"="请取降噪垫片2" ("Status")) -> ()  [unwired: 11 in]
                    n203 = call "Colour -电机.vi"("result"="等待", "colourRef"=w810) -> ()  [unwired: 9 in, 1 out]
                  }
                  frame "R563X" {
                    n204 = call "浮动通知.vi"("通知内容"="请取衬套2" ("Status")) -> ()  [unwired: 11 in]
                    n205 = call "Colour -电机.vi"("result"="等待", "colourRef"=w813) -> ()  [unwired: 9 in, 1 out]
                  }
                }
              }
              frame 10 {
                n206 = Index Array(array=w819, index=1 ("索引")) -> (element=w817:refnum<vi>)
                n207 = call "Colour -电机.vi"("result"="OK", "colourRef"=w817) -> ()  [unwired: 9 in, 1 out]
              }
              frame 11 {
                n208 = control-ref of="请取降噪块1"() -> (w822:refnum<vi>)
                n209 = call "浮动通知.vi"("通知内容"="请取降噪块1" ("Status")) -> ()  [unwired: 11 in]
                n210 = call "Colour -电机.vi"("result"="等待", "colourRef"=w822) -> ()  [unwired: 9 in, 1 out]
              }
              frame 12 {
                n211 = control-ref of="请取降噪块1"() -> (w823:refnum<vi>)
                n212 = call "Colour -电机.vi"("result"="OK", "colourRef"=w823) -> ()  [unwired: 9 in, 1 out]
              }
              frame 13 {
                n213 = global read "Global.vi" "产品型号"() -> (w828:string)
                n214 = case shown="\"R567X\"" w828 {
                  frame "假", Default {
                  }
                  frame "R567X" {
                  }
                }
                n215 = control-ref of="请取降噪块2"() -> (w827:refnum<vi>)
                n216 = call "浮动通知.vi"("通知内容"="请取降噪块2" ("Status")) -> ()  [unwired: 11 in]
                n217 = call "Colour -电机.vi"("result"="等待", "colourRef"=w827) -> ()  [unwired: 9 in, 1 out]
              }
              frame 14 {
                w829 = "OK" ("result")
                n218 = control-ref of="请取降噪块2"() -> (w832:refnum<vi>)
                n219 = control-ref of="请取锁紧块"() -> (w831:refnum<vi>)
                n220 = control-ref of="请安装推力滚针轴承"() -> (w830:refnum<vi>)
                n221 = call "Colour -电机.vi"("result"=w829, "colourRef"=w832) -> ()  [unwired: 9 in, 1 out]
                n222 = call "Colour -电机.vi"("result"=w829, "colourRef"=w831) -> ()  [unwired: 9 in, 1 out]
                n223 = call "Colour -电机.vi"("result"=w829, "colourRef"=w830) -> ()  [unwired: 9 in, 1 out]
              }
              frame 15 {
                n224 = control-ref of="请取锁紧块"() -> (w833:refnum<vi>)
                n225 = call "浮动通知.vi"("通知内容"="请取锁紧块" ("Status")) -> ()  [unwired: 11 in]
                n226 = call "Colour -电机.vi"("result"="等待", "colourRef"=w833) -> ()  [unwired: 9 in, 1 out]
              }
              frame 16 {
                n227 = shared-variable "我的电脑\\调节机构装配.lvlib\\设备状态"(u16 17 ("设备状态")) -> ()  [unwired: 1 in, 1 out]
                n228 = control-ref of="请取锁紧块"() -> (w837:refnum<vi>)
                n229 = call "Colour -电机.vi"("result"="OK", "colourRef"=w837) -> ()  [unwired: 9 in, 1 out]
              }
              frame 17 {
                n230 = control-ref of="请安装推力滚针轴承"() -> (w839:refnum<vi>)
                n231 = call "浮动通知.vi"("通知内容"="请安装轴承" ("Status")) -> ()  [unwired: 11 in]
                n232 = call "Colour -电机.vi"("result"="等待", "colourRef"=w839) -> ()  [unwired: 9 in, 1 out]
              }
              frame 18 {
                n233 = shared-variable "我的电脑\\调节机构装配.lvlib\\设备状态"(u16 19 ("设备状态")) -> ()  [unwired: 1 in, 1 out]
                n234 = control-ref of="请安装推力滚针轴承"() -> (w843:refnum<vi>)
                n235 = call "Colour -电机.vi"("result"="OK", "colourRef"=w843) -> ()  [unwired: 9 in, 1 out]
              }
              frame 19 {
                n236 = control-ref of="请安装挡片"() -> (w845:refnum<vi>)
                n237 = call "Colour -电机.vi"("result"="等待", "colourRef"=w845) -> ()  [unwired: 9 in, 1 out]
                n238 = call "浮动通知.vi"("通知内容"="请安装挡片" ("Status")) -> ()  [unwired: 11 in]
              }
              frame 20 {
                n239 = control-ref of="请安装挡片"() -> (w848:refnum<vi>)
                n240 = call "Colour -电机.vi"("result"="OK", "colourRef"=w848) -> ()  [unwired: 9 in, 1 out]
              }
              frame 21 {
                n241 = control-ref of="请安装锁紧螺母"() -> (w851:refnum<vi>)
                n242 = call "浮动通知.vi"("通知内容"="请安装锁紧螺母" ("Status")) -> ()  [unwired: 11 in]
                n243 = call "Colour -电机.vi"("result"="等待", "colourRef"=w851) -> ()  [unwired: 9 in, 1 out]
              }
              frame 22 {
                n244 = shared-variable "我的电脑\\调节机构装配.lvlib\\设备状态"(u16 23 ("设备状态")) -> ()  [unwired: 1 in, 1 out]
                n245 = control-ref of="请安装锁紧螺母"() -> (w854:refnum<vi>)
                n246 = call "Colour -电机.vi"("result"="OK", "colourRef"=w854) -> ()  [unwired: 9 in, 1 out]
              }
              frame 23 {
                n247 = call "浮动通知.vi"("通知内容"="请安装弹簧" ("Status")) -> ()  [unwired: 11 in]
                n248 = control-ref of="请安装弹簧"() -> (w856:refnum<vi>)
                n249 = call "Colour -电机.vi"("result"="等待", "colourRef"=w856) -> ()  [unwired: 9 in, 1 out]
              }
              frame 24 {
              }
              frame 25 {
                n250 = call "浮动通知.vi"("通知内容"="请拍照确认" ("Status")) -> ()  [unwired: 11 in]
                n251 = control-ref of="请安装弹簧"() -> (w859:refnum<vi>)
                n252 = call "Colour -电机.vi"("result"="OK", "colourRef"=w859) -> ()  [unwired: 9 in, 1 out]
                n253 = control-ref of="请拍照确认"() -> (w861:refnum<vi>)
                n254 = call "Colour -电机.vi"("result"="等待", "colourRef"=w861) -> ()  [unwired: 9 in, 1 out]
              }
              frame 30 {
                n255 = control-ref of="请拍照确认"() -> (w865:refnum<vi>)
                n256 = shared-variable "我的电脑\\调节机构装配.lvlib\\设备状态"(u16 200 ("设备状态")) -> ()  [unwired: 1 in, 1 out]
                n257 = call "Colour -电机.vi"("result"="OK", "colourRef"=w865) -> ()  [unwired: 9 in, 1 out]
              }
              frame 31 {
                n258 = control-ref of="请拍照确认"() -> (w867:refnum<vi>)
                n259 = call "Colour -电机.vi"("result"="NG", "colourRef"=w867) -> ()  [unwired: 9 in, 1 out]
                n260 = call "浮动通知.vi"("通知内容"="拍照不合格！" ("Status")) -> ()  [unwired: 11 in]
              }
              frame 35 {
                n261 = call "浮动通知.vi"("通知内容"="请安装固定螺栓1并确认扭矩！" ("Status")) -> ()  [unwired: 11 in]
              }
              frame 36 {
                n262 = Index Array(array=w878, index=1 ("索引")) -> (element=w877:refnum<vi>)
                n263 = Index Array(array=w878, index=4 ("索引")) -> (element=w872:refnum<vi>)
                n264 = call "Colour.vi"("result"="OK", "colourRef"=w877) -> ()  [unwired: 9 in, 1 out]
                n265 = call "Colour.vi"("result"="等待", "colourRef"=w872) -> ()  [unwired: 9 in, 1 out]
                n266 = call "浮动通知.vi"("通知内容"="请按启动拍照确认电机方向！" ("Status")) -> ()  [unwired: 11 in]
              }
              frame 40 {
                n267 = control-ref of="电机安装螺栓1扭矩确认"() -> (w879:refnum<vi>)
                n268 = call "Colour -电机.vi"("result"="等待", "colourRef"=w879) -> ()  [unwired: 9 in, 1 out]
                n269 = call "浮动通知.vi"("通知内容"="请安装固定螺栓1并确认扭矩！" ("Status")) -> ()  [unwired: 11 in]
              }
              frame 41 {
                n270 = flat-sequence {
                  frame #0 {
                    n271 = control-ref of="电机安装螺栓1扭矩确认"() -> (w882:refnum<vi>)
                    n272 = call "Colour -电机.vi"("result"="OK", "colourRef"=w882) -> ()  [unwired: 9 in, 1 out]
                  }
                  frame #1 {
                    n273 = local read "装配步骤"() -> (w886:T3)
                    n274 = local write "STEP3"("步骤" ("STEP3")) -> ()
                    n275 = Increment(x=w886) -> (x+1=w887:T3)
                    n276 = Wait (ms)(milliseconds to wait=u32 20 ("等待时间（毫秒）")) -> ()  [unwired: 1 out]
                    n277 = local write "装配步骤"(w887) -> ()
                  }
                }
              }
              frame 42 {
                n278 = control-ref of="电机安装螺栓2扭矩确认"() -> (w889:refnum<vi>)
                n279 = call "浮动通知.vi"("通知内容"="请安装固定螺栓2并确认扭矩！" ("Status")) -> ()  [unwired: 11 in]
                n280 = call "Colour -电机.vi"("result"="等待", "colourRef"=w889) -> ()  [unwired: 9 in, 1 out]
              }
              frame 43 {
                n281 = flat-sequence {
                  frame #0 {
                    n282 = control-ref of="电机安装螺栓2扭矩确认"() -> (w891:refnum<vi>)
                    n283 = call "Colour -电机.vi"("result"="OK", "colourRef"=w891) -> ()  [unwired: 9 in, 1 out]
                  }
                  frame #1 {
                    n284 = local read "装配步骤"() -> (w894:T3)
                    n285 = Increment(x=w894) -> (x+1=w895:T3)
                    n286 = local write "STEP3"("步骤" ("STEP3")) -> ()
                    n287 = local write "装配步骤"(w895) -> ()
                    n288 = Wait (ms)(milliseconds to wait=u32 20 ("等待时间（毫秒）")) -> ()  [unwired: 1 out]
                  }
                }
              }
              frame 44 {
                n289 = control-ref of="电机安装螺栓3扭矩确认"() -> (w898:refnum<vi>)
                n290 = call "浮动通知.vi"("通知内容"="请安装固定螺栓3并确认扭矩！" ("Status")) -> ()  [unwired: 11 in]
                n291 = call "Colour -电机.vi"("result"="等待", "colourRef"=w898) -> ()  [unwired: 9 in, 1 out]
              }
              frame 45 {
                n292 = flat-sequence {
                  frame #0 {
                    n293 = control-ref of="电机安装螺栓3扭矩确认"() -> (w900:refnum<vi>)
                    n294 = call "Colour -电机.vi"("result"="OK", "colourRef"=w900) -> ()  [unwired: 9 in, 1 out]
                  }
                  frame #1 {
                    n295 = local read "装配步骤"() -> (w903:T3)
                    n296 = Increment(x=w903) -> (x+1=w904:T3)
                    n297 = local write "STEP3"("步骤" ("STEP3")) -> ()
                    n298 = local write "装配步骤"(w904) -> ()
                    n299 = Wait (ms)(milliseconds to wait=u32 20 ("等待时间（毫秒）")) -> ()  [unwired: 1 out]
                  }
                }
              }
              frame 51 {
                n300 = call "浮动通知.vi"("通知内容"="请按启动按钮拍照确认！" ("Status")) -> ()  [unwired: 11 in]
              }
              frame 61 {
                n301 = Index Array(array=w913, index #1=3 ("索引")) -> (element #1=w911:refnum<vi>, element #2=w912:refnum<vi>)  [unwired: 1 in]
                n302 = call "Colour.vi"("result"="OK", "colourRef"=w911) -> ()  [unwired: 9 in, 1 out]
                n303 = call "Colour.vi"("result"="等待", "colourRef"=w912) -> ()  [unwired: 9 in, 1 out]
                n304 = call "浮动通知.vi"("通知内容"="请按启动拍照确认！" ("Status")) -> ()  [unwired: 11 in]
              }
              frame 70 {
                n305 = Index Array(array=w919, index #1=2 ("索引")) -> ()  [unwired: 1 in, 2 out]
                n306 = control-ref of="按启动按钮拍照确认"() -> (w915:refnum<vi>)
                n307 = control-ref of="电机安装螺栓3扭矩确认"() -> (w914:refnum<vi>)
                n308 = call "Colour -电机.vi"("result"="等待", "colourRef"=w915) -> ()  [unwired: 9 in, 1 out]
                n309 = call "Colour -电机.vi"("result"="OK", "colourRef"=w914) -> ()  [unwired: 9 in, 1 out]
              }
              frame 80 {
                n310 = control-ref of="按启动按钮拍照确认"() -> (w921:refnum<vi>)
                n311 = call "Colour -电机.vi"("result"="NG", "colourRef"=w921) -> ()  [unwired: 9 in, 1 out]
              }
              frame 81 {
                n312 = flat-sequence {
                  frame #0 {
                    n313 = control-ref of="按启动按钮拍照确认"() -> (w923:refnum<vi>)
                    n314 = call "Colour -电机.vi"("result"="OK", "colourRef"=w923) -> ()  [unwired: 9 in, 1 out]
                  }
                  frame #1 {
                    n315 = local read "装配步骤"() -> (w926:T3)
                    n316 = Increment(x=w926) -> (x+1=w927:T3)
                    n317 = Wait (ms)(milliseconds to wait=u32 20 ("等待时间（毫秒）")) -> ()  [unwired: 1 out]
                    n318 = local write "STEP3"("步骤" ("STEP3")) -> ()
                    n319 = local write "装配步骤"(w927) -> ()
                  }
                }
              }
              frame 90 {
                n320 = Index Array(array=w931, index #1=3 ("索引")) -> ()  [unwired: 1 in, 2 out]
                n321 = control-ref of="涂色标"() -> (w929:refnum<vi>)
                n322 = call "浮动通知.vi"("通知内容"="请给固定螺栓涂色标！" ("Status")) -> ()  [unwired: 11 in]
                n323 = call "Colour -电机.vi"("result"="等待", "colourRef"=w929) -> ()  [unwired: 9 in, 1 out]
              }
              frame 91 {
                n324 = flat-sequence {
                  frame #0 {
                    n325 = control-ref of="涂色标"() -> (w933:refnum<vi>)
                    n326 = call "Colour -电机.vi"("result"="OK", "colourRef"=w933) -> ()  [unwired: 9 in, 1 out]
                  }
                  frame #1 {
                    n327 = local read "装配步骤"() -> (w937:T3)
                    n328 = Increment(x=w937) -> (x+1=w938:T3)
                    n329 = local write "STEP3"("步骤" ("STEP3")) -> ()
                    n330 = Wait (ms)(milliseconds to wait=u32 20 ("等待时间（毫秒）")) -> ()  [unwired: 1 out]
                    n331 = local write "装配步骤"(w938) -> ()
                  }
                }
              }
              frame 100 {
                n332 = Index Array(array=w941, index #1=4 ("索引")) -> ()  [unwired: 1 in, 2 out]
                n333 = control-ref of="安装扎带并取走工件"() -> (w940:refnum<vi>)
                n334 = call "Colour -电机.vi"("result"="等待", "colourRef"=w940) -> ()  [unwired: 9 in, 1 out]
                n335 = call "浮动通知.vi"("通知内容"="请安装轧带并取走工件" ("Status")) -> ()  [unwired: 11 in]
              }
              frame 101 {
                n336 = Index Array(array=w944, index #1=5 ("索引")) -> ()  [unwired: 1 in, 2 out]
                n337 = flat-sequence {
                  frame #0 {
                    n338 = control-ref of="安装扎带并取走工件"() -> (w947:refnum<vi>)
                    n339 = call "浮动通知.vi"("通知内容"="完成！" ("Status")) -> ()  [unwired: 11 in]
                    n340 = call "Colour -电机.vi"("result"="OK", "colourRef"=w947) -> ()  [unwired: 9 in, 1 out]
                  }
                  frame #1 {
                    n341 = local read "装配步骤"() -> (w951:T3)
                    n342 = Increment(x=w951) -> (x+1=w950:T3)
                    n343 = local write "STEP3"("步骤" ("STEP3")) -> ()
                    n344 = Wait (ms)(milliseconds to wait=u32 20 ("等待时间（毫秒）")) -> ()  [unwired: 1 out]
                    n345 = local write "装配步骤"(w950) -> ()
                  }
                }
              }
              frame 128 {
                n346 = call "浮动通知.vi"("通知内容"="复位中……" ("Status")) -> ()  [unwired: 11 in]
                n347 = global read "Global.vi" "电机程序自动"() -> (w954:refnum<vi>)
                n348 = property class="Bool"(reference=w954, "Value"=FALSE) -> ()  [unwired: 1 in, 2 out]
              }
              frame 200 {
                n349 = global read "Global1.vi" "联机模式"() -> (w956:enum16{"单机", "追溯"})
                n350 = Wait (ms)(milliseconds to wait=u32 500 ("等待时间（毫秒）")) -> ()  [unwired: 1 out]
                n351 = case shown="\"追溯\"" w956 {
                  frame "单机", Default {
                    n352 = call "浮动通知.vi"("通知内容"="产品合格！" ("Status")) -> ()  [unwired: 11 in]
                    n353 = Wait (ms)(milliseconds to wait=u32 200 ("等待时间（毫秒）")) -> ()  [unwired: 1 out]
                    n354 = local write "STEP3"("初始化" ("STEP3")) -> ()
                    n355 = shared-variable "我的电脑\\调节机构装配.lvlib\\设备状态"(u16 6 ("设备状态")) -> ()  [unwired: 1 in, 1 out]
                  }
                  frame "追溯" {
                    n356 = global write "Global1.vi" "装配结果"("OK" ("装配结果")) -> ()
                    n357 = call "浮动通知.vi"("通知内容"="产品合格！" ("Status")) -> ()  [unwired: 11 in]
                    n358 = global read "Global1.vi" "联机模式"() -> (w963:enum16{"单机", "追溯"})
                    n359 = case shown="\"追溯\"" w963 {
                      tunnel: ["等待" "录入数据库" ("STEP3")] -> w964
                      frame "单机", Default {
                        n360 = local write "装配步骤"(T3."降噪片1" ("装配步骤")) -> ()
                      }
                      frame "追溯" {
                      }
                    }
                    n361 = local write "STEP3"(w964) -> ()
                  }
                }
              }
              frame 201 {
                n362 = global read "Global.vi" "检测结果"() -> (w970:refnum<vi>)
                n363 = call "Colour.vi"("result"="NG", "colourRef"=w970) -> ()  [unwired: 9 in, 1 out]
                n364 = call "浮动通知.vi"("通知内容"="产品不合格！" ("Status")) -> ()  [unwired: 11 in]
              }
              frame 999 {
                n365 = Index Array(array=w974, index #1=0 ("索引")) -> (element #1=w981:refnum<vi>, element #2=w982:refnum<vi>, element #3=w975:refnum<vi>, element #4=w972:refnum<vi>)  [unwired: 3 in]
                n366 = call "Colour.vi"("result"="", "colourRef"=w975) -> ()  [unwired: 9 in, 1 out]
                n367 = call "Colour.vi"("result"="", "colourRef"=w972) -> ()  [unwired: 9 in, 1 out]
                n368 = call "Colour.vi"("result"="NG", "colourRef"=w982) -> ()  [unwired: 9 in, 1 out]
                n369 = call "Colour.vi"("result"="OK", "colourRef"=w981) -> ()  [unwired: 9 in, 1 out]
                n370 = call "浮动通知.vi"("通知内容"="请重新安装固定螺栓！" ("Status")) -> ()  [unwired: 11 in]
              }
              frame 1024 {
                n371 = call "浮动通知.vi"("通知内容"="急停！" ("Status")) -> ()  [unwired: 11 in]
                n372 = global read "Global.vi" "电机程序自动"() -> (w984:refnum<vi>)
                n373 = property class="Bool"(reference=w984, "Value"=FALSE) -> ()  [unwired: 1 in, 2 out]
              }
              frame 3721 {
                n374 = local write "STEP3"("不合格锁定" ("STEP")) -> ()
                n375 = call "浮动通知.vi"("通知内容"="产品不合格程序锁定！" ("Status")) -> ()  [unwired: 11 in]
              }
              frame 3722 {
                n376 = global read "Global.vi" "电机程序自动"() -> (w989:refnum<vi>)
                n377 = call "浮动通知.vi"("通知内容"="授权成功，请复位！" ("Status")) -> ()  [unwired: 11 in]
                n378 = property class="Bool"(reference=w989, "Value"=FALSE) -> ()  [unwired: 1 in, 2 out]
              }
              frame 3723 {
                n379 = call "浮动通知.vi"("通知内容"="请取出不合格产品并摆放至不合格品区！" ("Status")) -> ()  [unwired: 11 in]
              }
              frame Default {
              }
            }
          }
          frame "录入数据库" {
            n380 = stacked-sequence {
              frame #0 {
                n381 = Get Date/Time String(date format (0)=enum16{"short", "long", "abbreviated"}."short" ("日期格式(0)"), want seconds? (F)=FALSE ("需要秒？(F)")) -> (date string=w1002:string, time string=w1003:string)  [unwired: 1 in]
                n382 = global read "Global1.vi" "DEVICE_ID"() -> (w1006:string)
                n383 = global read "Global1.vi" "USER_ID"() -> (w1004:string)
                n384 = global read "Global1.vi" "CODE_ID"() -> (w1005:string)
                n385 = global read "Global1.vi" "装配结果"() -> (w997:string)
                n386 = Concatenate Strings(w1002, " " ("字符串"), w1003) -> (w998:string)
                n387 = global read "Global1.vi" "联机模式"() -> (w992:enum16{"单机", "追溯"})
                n388 = Decimal String To Number(string=w1006, default (0L)=i64 0 ("默认(0 I32)")) -> (number=w995:i64)  [unwired: 1 in, 1 out]
                n389 = Decimal String To Number(string=w1004, default (0L)=i64 0 ("默认(0 I32)")) -> (number=w994:i64)  [unwired: 1 in, 1 out]
                n390 = Decimal String To Number(string=w1005, default (0L)=i64 0 ("默认(0 I32)")) -> (number=w993:i64)  [unwired: 1 in, 1 out]
                n391 = Search and Replace String(replace all?=TRUE ("替换全部？(F)"), input string=w998, search string="/" ("替换字符串(\"\")"), replace string="-" ("替换字符串(\"\")")) -> (result string=w996:string)  [unwired: 4 in, 3 out]
                n392 = Bundle(w995, w994, w993, "装配结果"=w997, "result string"=w996) -> (w1018:T4)  [unwired: 1 in]
                n393 = call "GetSQLstring.vi"("联机模式"=w992) -> ("错误输出"=w1015:errorcluster, "连接字符串"=w1014:string)  [unwired: 9 in]
                n394 = Build Array(w1018) -> (w1019:T5)
                n395 = call-poly <vilib>:"DB Tools Open Connection.vi"("error in (no error)"=w1015, "connection information"=w1014) -> ("error out"=w1013:errorcluster, "connection reference"=w1016:T6)  [unwired: 6 in]
                n396 = for {
                  tunnel: w1019 -> [w1024] mode=indexing
                  tunnel: w1016 -> [w1022]
                  shift-right: [w1020] -> w1017
                  shift-left: w1013 -> [w1027]
                  w1023 = string[] ["DEVICE_ID", "USER_ID", "CODE_ID", "RESULT_VALUE", "RESULT_TIME"] ("columns")
                  w1025 = "Result" ("table")
                  n397 = call <vilib>:"DB Tools Insert Data.vi"("data"=w1024, "error in (no error)"=w1027, "columns"=w1023, "table"=w1025, "connection reference"=w1022) -> ("error out"=w1026:errorcluster, "connection reference out"=w1021:T6)  [unwired: 5 in]
                  n398 = case shown="错误" w1026 {
                    selector: w1026 -> [w1028 w1049]
                    tunnel: w1023 -> [_ w1046]
                    tunnel: w1021 -> [w1029 w1038]
                    tunnel: w1025 -> [_ w1050]
                    tunnel: w1024 -> [_ w1042]
                    tunnel: [w1029 w1037] -> _
                    tunnel: [w1028 w1036] -> w1020
                    frame No Error {
                    }
                    frame Error {
                      n399 = Array Subset(array=w1046, index=3 ("长度"), length=2 ("长度")) -> (w1047:string[])
                      n400 = Unbundle(w1042) -> (w1031:i64, w1034:i64, "装配结果"=w1041:string, "result string"=w1040:string)  [unwired: 1 out]
                      n401 = Number To Decimal String(number=w1034) -> (decimal integer string=w1035:string)  [unwired: 1 in]
                      n402 = Number To Decimal String(number=w1031) -> (decimal integer string=w1030:string)  [unwired: 1 in]
                      n403 = Concatenate Strings("WHERE CODE_ID =" ("condition"), w1035, "AND DEVICE_ID = ", w1030) -> (w1043:string)
                      n404 = Bundle("装配结果"=w1041, "result string"=w1040) -> (w1039:cluster{"装配结果":string, "result string":string})  [unwired: 1 in]
                      n405 = call <vilib>:"Clear Errors.vi"("error in (no error)"=w1049) -> ("error out"=w1048:errorcluster)  [unwired: 5 in, 1 out]
                      n406 = call <vilib>:"DB Tools Update Data.vi"("condition"=w1043, "data"=w1039, "error in (no error)"=w1048, "columns"=w1047, "table"=w1050, "connection reference"=w1038) -> ("error out"=w1036:errorcluster, "connection reference out"=w1037:T6)  [unwired: 4 in]
                    }
                  }
                }
                n407 = call <vilib>:"Simple Error Handler.vi"("error in (no error)"=w1017) -> ()  [unwired: 4 in, 5 out]
              }
              frame #1 {
                (unwired) enum16{"单机", "联网"}."联网" ("联机模式")
                n408 = global read "Global1.vi" "管柱码"() -> (w1051:string)
                n409 = global read "Global1.vi" "CODE_ID"() -> (w1052:string)
                n410 = Format Into String(format string="UPDATE\ndbo.[Code]\nSET dbo.[Code].CODE_MAIN = '%s'\n\nWHERE\ndbo.[Code].CODE_ID = %s\n" ("格式字符串"), w1051, w1052) -> (resulting string=w1054:string)  [unwired: 2 in, 1 out]
                n411 = call "SQL_query.vi"("SQL query"=w1054) -> ()  [unwired: 2 in, 3 out]
              }
              frame #2 {
                n412 = call "浮动通知.vi"("通知内容"="数据录入成功！" ("Status")) -> ()  [unwired: 11 in]
                n413 = local write "装配步骤"(T3."降噪片1" ("装配步骤")) -> ()
                n414 = shared-variable "我的电脑\\调节机构装配.lvlib\\设备状态"(i16 6 ("设备状态")) -> ()  [unwired: 1 in, 1 out]
                n415 = local write "STEP3"("初始化" ("STEP")) -> ()
                n416 = Wait (ms)(milliseconds to wait=u32 500 ("等待时间（毫秒）")) -> ()  [unwired: 1 out]
              }
            }
          }
          frame "不合格锁定" {
            n417 = call "临时授权.vi"() -> ("授权成功"=w1061:bool)  [unwired: 11 in]
            n418 = case shown="真" w1061 {
              frame False {
              }
              frame True {
                (unwired) i16 3722 ("设备状态")
                n419 = local write "STEP3"("报表" ("STEP")) -> ()
              }
            }
            n420 = Wait (ms)(milliseconds to wait=u32 100 ("等待时间（毫秒）")) -> ()  [unwired: 1 out]
          }
          frame "报表" {
            n421 = call "浮动通知.vi"("通知内容"="报表生成中" ("Status")) -> ()  [unwired: 11 in]
            n422 = shared-variable "我的电脑\\Global.lvlib\\工位追溯码"() -> (w1072:string)  [unwired: 1 in, 1 out]
            n423 = Index Array(array="判定结果", index (col)=1 ("禁用的索引 (列)")) -> (element=w1067:bool[])  [unwired: 1 in]
            n424 = And Array Elements(Boolean array=w1067) -> (logical AND=w1064:bool)
            n425 = shared-variable "我的电脑\\Global.lvlib\\联机模式"() -> (w1069:i16)  [unwired: 1 in, 1 out]
            n426 = call "Report_A170316-11.vi"("文件重命名"=TRUE, "文件名称"=w1072, "布尔数组"="判定结果") -> ("error out"=w1070:errorcluster)  [unwired: 8 in]
            n427 = case shown="真" w1064 {
              frame False {
              }
              frame True {
              }
            }
            n428 = case shown="0, 默认" w1069 {
              tunnel: w1070 -> [_ w1075]
              frame 0, Default {
              }
              frame 1 {
                n429 = call "上传数据库.vi"("错误输入"=w1075) -> ()  [unwired: 10 in, 1 out]
              }
            }
            n430 = shared-variable "我的电脑\\调节机构装配.lvlib\\设备状态"() -> (w1063:u16)  [unwired: 1 in, 1 out]
            n431 = case shown="3721..3723" w1063 {
              frame Default {
                n432 = local write "STEP3"("初始化" ("STEP")) -> ()
              }
              frame 3721..3723 {
                n433 = local write "STEP3"("等待" ("STEP")) -> ()
              }
            }
          }
          frame "步骤" {
            n434 = case shown="\"降噪片1\", 默认" "装配步骤" {
              selector: "装配步骤" -> [w1079 _]
              tunnel: [w1078 "等待"] -> w1076
              frame "降噪片1", Default {
                n435 = global read "Global.vi" "手柄安装步骤"() -> (w1081:bool[])
                n436 = Index Array(array=w1081, index=w1079) -> (element=w1080:bool)
                n437 = case shown="真" w1080 {
                  tunnel: w1079 -> [_ w1086]
                  tunnel: ["步骤" w1085] -> w1078
                  frame False {
                    n438 = local read "装配步骤"() -> (w1084:T3)
                    n439 = Increment(x=w1084) -> (x+1=w1083:T3)
                    n440 = local write "装配步骤"(w1083) -> ()
                  }
                  frame True {
                    n441 = case shown="\"轴承拍照\"" w1086 {
                      tunnel: ["等待" "等待" "等待" "等待" "等待" "等待" "等待" "等待" "等待" "等待"] -> w1085
                      frame "降噪片1", Default {
                        n442 = shared-variable "我的电脑\\调节机构装配.lvlib\\设备状态"(u16 7 ("设备状态")) -> ()  [unwired: 1 in, 1 out]
                      }
                      frame "降噪片2" {
                        n443 = shared-variable "我的电脑\\调节机构装配.lvlib\\设备状态"(i16 9 ("设备状态")) -> ()  [unwired: 1 in, 1 out]
                      }
                      frame "降噪块1" {
                        n444 = shared-variable "我的电脑\\调节机构装配.lvlib\\设备状态"(u16 11 ("设备状态")) -> ()  [unwired: 1 in, 1 out]
                      }
                      frame "降噪块2" {
                        n445 = shared-variable "我的电脑\\调节机构装配.lvlib\\设备状态"(u16 13 ("设备状态")) -> ()  [unwired: 1 in, 1 out]
                      }
                      frame "锁紧块" {
                      }
                      frame "滚针轴承" {
                      }
                      frame "垫片" {
                        n446 = shared-variable "我的电脑\\调节机构装配.lvlib\\设备状态"(u16 15 ("设备状态")) -> ()  [unwired: 1 in, 1 out]
                      }
                      frame "锁紧螺母" {
                      }
                      frame "弹簧" {
                        n447 = shared-variable "我的电脑\\调节机构装配.lvlib\\设备状态"(u16 17 ("设备状态")) -> ()  [unwired: 1 in, 1 out]
                      }
                      frame "轴承拍照" {
                        n448 = shared-variable "我的电脑\\调节机构装配.lvlib\\设备状态"(u16 20 ("设备状态")) -> ()  [unwired: 1 in, 1 out]
                      }
                    }
                  }
                }
              }
              frame "完成" {
                n449 = shared-variable "我的电脑\\调节机构装配.lvlib\\设备状态"(u16 200 ("设备状态")) -> ()  [unwired: 1 in, 1 out]
              }
            }
            n450 = local write "STEP3"(w1076) -> ()
          }
        }
        n451 = global read "Global.vi" "程序关闭"() -> (w633:bool)
      }
      n452 = disable-structure shown="禁用" {
        frame Disabled {
          n453 = while {
            stop <- w53 stop-if-true
            n454 = Wait Until Next ms Multiple(millisecond multiple=u32 10 ("毫秒倍数")) -> ()  [unwired: 1 out]
            n455 = case shown="\"自动\"" "STEP2" {
              frame "等待", Default {
                n456 = local write "STEP2"("自动" ("STEP")) -> ()
              }
              frame "手动" {
              }
              frame "初始化" {
                n457 = stacked-sequence {
                  frame #0 {
                    w179 = enum16{"录入", "清空"}."清空" ("功能")
                    n458 = global read "Global.vi" "安装支架生产数量"() -> (w171:refnum<vi>)
                    n459 = shared-variable "我的电脑\\Global.lvlib\\工位追溯码"("" ("传感器码")) -> ()  [unwired: 1 in, 1 out]
                    n460 = call "物料信息录入.vi"("功能"=w179) -> ("错误输出"=w178:errorcluster)  [unwired: 14 in]
                    n461 = call "质量信息录入.vi"("功能"=w179, "错误输入（无错误）"=w178) -> ("错误输出"=w180:errorcluster)  [unwired: 13 in]
                    n462 = property class="Num"(reference=w171, "Value"=0 ("磨合次数")) -> ()  [unwired: 1 in, 2 out]
                    n463 = call "不合格信息录入.vi"("功能"=w179, "错误输入（无错误）"=w180) -> ()  [unwired: 13 in, 1 out]
                    n464 = global read "Global.vi" "ECU自动"() -> (w176:refnum<vi>)
                    n465 = global read "Global.vi" "检测结果"() -> (w174:refnum<vi>)
                    n466 = property class="Bool (严格)"(reference=w176, "Value"=TRUE) -> ()  [unwired: 1 in, 2 out]
                    n467 = shared-variable "我的电脑\\A17031611.lvlib\\设备状态2"(i16 6 ("设备状态")) -> ()  [unwired: 1 in, 1 out]
                    n468 = call "Colour.vi"("result"="", "colourRef"=w174) -> ()  [unwired: 9 in, 1 out]
                  }
                  frame #1 {
                    n469 = local write "ECU步骤"(T2."控制器安装螺栓1" ("ECU步骤")) -> ()
                  }
                  frame #2 {
                    n470 = local write "STEP2"("等待" ("STEP2")) -> ()
                  }
                }
              }
              frame "扫主码" {
                n471 = stacked-sequence {
                  frame #0 {
                    w184 = "请扫ECU工位主码！" ("提示信息")
                    n472 = call "浮动通知2.vi"("通知内容"=w184) -> ()  [unwired: 11 in]
                    n473 = call "输入框.vi"("提示信息"=w184) -> ("条形码输出"=w185:string)
                    n474 = case shown="\"\", 默认" w185 {
                      selector: w185 -> [w186 _]
                      tunnel: [w187 "手动"] -> w183
                      frame "", Default {
                        n475 = shared-variable "我的电脑\\Global.lvlib\\工位追溯码_ECU"(w186) -> ()  [unwired: 1 in, 1 out]
                        n476 = global write "Global1.vi" "工位追溯码_ECU"(w186) -> ()
                        n477 = global read "Global1.vi" "联机模式"() -> (w188:enum16{"单机", "追溯"})
                        n478 = case shown="\"追溯\"" w188 {
                          tunnel: w186 -> [_ w191]
                          tunnel: ["控制器扫码" ("State(s) in Front (\"\")") w190] -> w187
                          frame "单机", Default {
                          }
                          frame "追溯" {
                            n479 = stacked-sequence {
                              tunnel: w191 -> [w192 _ _]
                              tunnel: [_ _ w212] -> w190
                              frame #0 {
                                n480 = global read "Global1.vi" "PRODUCT_ID_ECU"() -> (w196:string)
                                n481 = Format Into String "格式化写入字符串"(format string="SELECT\ndbo.[Code].CODE_ID\nFROM\ndbo.[Code]\nWHERE\ndbo.[Code].CODE_MAIN = '%s'\nAND\ndbo.[Code].PRODUCT_ID = %s\n" ("格式字符串"), w192, w196) -> (resulting string=w198:string)  [unwired: 2 in, 1 out]
                                n482 = call "SQL_query.vi"("SQL query"=w198, "联机模式"=enum16{"单机", "联网"}."联网") -> ("data"=w201:string[][])  [unwired: 1 in, 2 out]
                                n483 = Index Array(array=w201, index (row)=0 ("索引 (行)")) -> (element=w200:string[])  [unwired: 1 in]
                                n484 = Index Array(array=w200, index=0 ("索引")) -> (element=w193:string)
                                n485 = global write "Global1.vi" "CODE_ID_ECU"(w193) -> ()
                              }
                              frame #1 {
                                n486 = global read "Global1.vi" "前序DEVICE_ID_ECU"() -> (w202:string)
                                n487 = global read "Global1.vi" "CODE_ID_ECU"() -> (w203:string)
                                n488 = Format Into String(format string="SELECT\ndbo.[Result].RESULT_VALUE\nFROM\ndbo.[Result]\nWHERE\ndbo.[Result].DEVICE_ID = %s\nAND\ndbo.[Result].CODE_ID = %s\n" ("格式字符串"), w202, w203) -> (resulting string=w205:string)  [unwired: 2 in, 1 out]
                                n489 = call "SQL_query.vi"("SQL query"=w205, "联机模式"=enum16{"单机", "联网"}."联网") -> ("data"=w211:string[][])  [unwired: 1 in, 2 out]
                                n490 = Index Array(array=w211, index (row)=0 ("索引 (行)")) -> (element=w210:string[])  [unwired: 1 in]
                                n491 = Index Array(array=w210, index=0 ("索引")) -> (element=w204:string)
                                n492 = local write "前序OK？_ECU"(w204) -> ()
                              }
                              frame #2 {
                                n493 = local read "前序OK？_ECU"() -> (w213:string)
                                n494 = case shown="\"OK\"" w213 {
                                tunnel: ["控制器扫码" "自动" "自动"] -> w212
                                frame "OK" {
                                n495 = global read "Global.vi" "ECU前序显示字"() -> (w216:refnum<vi>)
                                n496 = global read "Global1.vi" "ECU上序状态"() -> (w215:refnum<vi>)
                                n497 = property class="Str"(reference=w216, "Value"="OK" ("值")) -> ()  [unwired: 1 in, 2 out]
                                n498 = call "Colour -ECU.vi"("result"="OK", "colourRef"=w215) -> ()  [unwired: 9 in, 1 out]
                                }
                                frame Default {
                                n499 = global read "Global1.vi" "ECU上序状态"() -> (w222:refnum<vi>)
                                n500 = Wait (ms)(milliseconds to wait=u32 3000 ("等待时间（毫秒）")) -> ()  [unwired: 1 out]
                                n501 = call "浮动通知2.vi"("通知内容"="ECU工位上序漏序！" ("Status")) -> ()  [unwired: 11 in]
                                n502 = global read "Global.vi" "ECU前序显示字"() -> (w219:refnum<vi>)
                                n503 = call "Colour.vi"("result"="等待", "colourRef"=w222) -> ()  [unwired: 9 in, 1 out]
                                n504 = shared-variable "我的电脑\\A17031611.lvlib\\设备状态2"(i16 6 ("设备状态控制字")) -> ()  [unwired: 1 in, 1 out]
                                n505 = property class="Str"(reference=w219, "Value"="漏序" ("值")) -> ()  [unwired: 1 in, 2 out]
                                }
                                frame "NG" {
                                n506 = Wait (ms)(milliseconds to wait=u32 3000 ("等待时间（毫秒）")) -> ()  [unwired: 1 out]
                                n507 = global read "Global1.vi" "ECU上序状态"() -> (w228:refnum<vi>)
                                n508 = call "浮动通知2.vi"("通知内容"="上序生产结果不合格！" ("Status")) -> ()  [unwired: 11 in]
                                n509 = global read "Global.vi" "ECU前序显示字"() -> (w230:refnum<vi>)
                                n510 = call "Colour -ECU.vi"("result"="NG", "colourRef"=w228) -> ()  [unwired: 9 in, 1 out]
                                n511 = shared-variable "我的电脑\\A17031611.lvlib\\设备状态2"(i16 6 ("设备状态控制字")) -> ()  [unwired: 1 in, 1 out]
                                n512 = property class="Str"(reference=w230, "Value"="NG" ("值")) -> ()  [unwired: 1 in, 2 out]
                                }
                                }
                              }
                            }
                          }
                        }
                      }
                      frame "exit" {
                      }
                    }
                    n513 = local write "STEP2"(w183) -> ()
                  }
                  frame #1 {
                    n514 = Wait (ms)(milliseconds to wait=u32 100 ("等待时间（毫秒）")) -> ()  [unwired: 1 out]
                  }
                }
              }
              frame "控制器扫码" {
                n515 = stacked-sequence {
                  frame #0 {
                    w237 = "请扫请控制器码！！" ("提示信息")
                    n516 = call "输入框.vi"("提示信息"=w237) -> ("条形码输出"=w238:string)
                    n517 = call "浮动通知2.vi"("通知内容"=w237) -> ()  [unwired: 11 in]
                    n518 = case shown="\"\", 默认" w238 {
                      selector: w238 -> [w244 _]
                      tunnel: [w247 "手动"] -> w239
                      frame "", Default {
                        n519 = global read "Global.vi" "硬件版本号"() -> (w240:string)
                        n520 = global write "Global1.vi" "控制器码"(w244) -> ()
                        n521 = shared-variable "我的电脑\\Global.lvlib\\控制器码"(w244) -> ()  [unwired: 1 in, 1 out]
                        n522 = xnode "匹配正则表达式"("输入字符串"=w244, "正则表达式"="-") -> ("匹配之前"=w242:string)  [unwired: 4 in, 4 out]
                        n523 = call <vilib>:"Trim Whitespace.vi"("string"=w242) -> ("trimmed string"=w245:string)  [unwired: 1 in]
                        n524 = call <vilib>:"Trim Whitespace.vi"("string"=w240) -> ("trimmed string"=w246:string)  [unwired: 1 in]
                        n525 = Equal?(x=w245, y=w246) -> (x = y?=w241:bool)
                        n526 = case shown="真" w241 {
                          tunnel: ["控制器扫码" ("State(s) in Front (\"\")") w367] -> w247
                          frame False {
                            w365 = 0 items=["OK", "OKCancel", "AbortRetryIgnore", "YesNoCancel", "YesNo", "RetryCancel"] ("buttons")
                            w366 = 16 items=["None"=0, "Hand, Error, Stop"=16, "Question"=32, "Exclamation, Warning"=48, "Asterisk, Information"=64] ("icon")
                            n527 = call "信息框（标题、文本、图标）.vi"("icon"=w366, "buttons"=w365, "caption"="控制器混料", "text"="混料请核对控制器!") -> ()  [unwired: 6 in, 2 out]
                          }
                          frame True {
                            n528 = global read "Global1.vi" "联机模式"() -> (w368:enum16{"单机", "追溯"})
                            n529 = case shown="\"单机\", 默认" w368 {
                              tunnel: ["步骤" ("State(s) in Front (\"\")") "步骤"] -> w367
                              frame "单机", Default {
                                n530 = global read "Global.vi" "安装支架生产数量"() -> (w372:refnum<vi>)
                                n531 = property class="Num"(reference=w372) -> (reference out=w373:refnum<vi>, error out=w374:errorcluster, "Value"=w375:variant)  [unwired: 1 in]
                                n532 = Variant To Data(type=u32 0, Variant=w375) -> (data=w376:u32)  [unwired: 1 in, 1 out]
                                n533 = Increment(x=w376) -> (x+1=w377:u32)
                                n534 = property class="Num"(reference=w373, error in=w374, "Value"=w377) -> ()  [unwired: 2 out]
                                n535 = Wait (ms)(milliseconds to wait=u32 10 ("等待时间（毫秒）")) -> ()  [unwired: 1 out]
                              }
                              frame "追溯" {
                                n536 = global read "Global.vi" "安装支架生产数量"() -> (w379:refnum<vi>)
                                n537 = property class="Num"(reference=w379) -> (reference out=w380:refnum<vi>, error out=w381:errorcluster, "Value"=w382:variant)  [unwired: 1 in]
                                n538 = Variant To Data "变体至数据转换"(type=u32 0, Variant=w382) -> (data=w383:u32)  [unwired: 1 in, 1 out]
                                n539 = Increment(x=w383) -> (x+1=w384:u32)
                                n540 = property class="Num"(reference=w380, error in=w381, "Value"=w384) -> ()  [unwired: 2 out]
                              }
                            }
                          }
                        }
                      }
                      frame "exit" {
                      }
                    }
                    n541 = local write "STEP2"(w239) -> ()
                  }
                  frame #1 {
                    n542 = Wait (ms)(milliseconds to wait=u32 100 ("等待时间（毫秒）")) -> ()  [unwired: 1 out]
                  }
                }
              }
              frame "自动" {
                # "3=41\n2=42\n1=43\n0=45"
                # "4=31\n3=32\n2=33\n1=34\n0=35"
                n543 = shared-variable "我的电脑\\A17031611.lvlib\\安装支架螺栓2"() -> (w388:u16)  [unwired: 1 in, 1 out]
                n544 = shared-variable "我的电脑\\A17031611.lvlib\\安装支架螺栓数"() -> (w389:u16)  [unwired: 1 in, 1 out]
                n545 = shared-variable "我的电脑\\A17031611.lvlib\\设备状态2"() -> (w390:i16)  [unwired: 1 in, 1 out]
                n546 = global read "A170316-11.vi" "安装支架LED"() -> (w391:refnum<vi>[])
                n547 = case shown="44" w390 {
                  tunnel: w391 -> [_ _ _ _ _ w395 _ w403 _ _ _ _ _ _ _ _ _ _ _ _ _ _ _ w469 w471 _ _ w487 w490 w497 _ _ w524 _ _ _ _]
                  tunnel: w389 -> [_ _ _ _ _ _ _ w404 _ _ _ _ _ _ _ _ _ _ _ _ _ _ _ _ _ _ _ _ _ _ _ _ _ _ _ _ _]
                  tunnel: w388 -> [_ _ _ _ _ _ _ _ _ _ _ _ _ _ _ _ _ _ _ _ _ _ _ _ _ _ _ _ _ _ _ _ _ _ _ _ _]
                  frame Default {
                  }
                  frame -128 {
                    n548 = global read "Global.vi" "ECU自动"() -> (w393:refnum<vi>)
                    n549 = property class="Bool (严格)"(reference=w393, "Value"=FALSE) -> ()  [unwired: 1 in, 2 out]
                  }
                  frame 5 {
                    (unwired) "ECU工位复位完成！" ("Status")
                  }
                  frame 6 {
                    n550 = call "浮动通知2.vi"("通知内容"="请按启动确认扫ECU工位主码") -> ()  [unwired: 11 in]
                  }
                  frame 0 {
                    (unwired) "手动状态！" ("Status")
                  }
                  frame 7 {
                    n551 = for {
                      tunnel: w395 -> [w402] mode=indexing
                      n552 = call "Colour -ECU.vi"("result"="", "colourRef"=w402) -> ()  [unwired: 9 in, 1 out]
                    }
                    n553 = global read "Global.vi" "ECU结果显示"() -> (w397:refnum<vi>)
                    n554 = property class="Str"(reference=w397, "Value"="..." ("结果显示")) -> (reference out=w398:refnum<vi>)  [unwired: 1 in, 1 out]
                    n555 = property class="Str"(reference=w398, "Text.TextColor"=u32 16776960) -> ()  [unwired: 1 in, 2 out]
                    n556 = local write "STEP2"("扫主码" ("STEP2")) -> ()
                  }
                  frame 9 {
                  }
                  frame 10 {
                    n557 = case shown="2" w404 {
                      tunnel: w403 -> [_ _ _ _ _]
                      frame 0, Default {
                        n558 = shared-variable "我的电脑\\A17031611.lvlib\\设备状态2"(i16 35 ("设备状态")) -> ()  [unwired: 1 in, 1 out]
                      }
                      frame 1 {
                        n559 = shared-variable "我的电脑\\A17031611.lvlib\\设备状态2"(i16 34 ("设备状态")) -> ()  [unwired: 1 in, 1 out]
                      }
                      frame 2 {
                        n560 = shared-variable "我的电脑\\A17031611.lvlib\\设备状态2"(i16 33 ("设备状态")) -> ()  [unwired: 1 in, 1 out]
                      }
                      frame 3 {
                        n561 = shared-variable "我的电脑\\A17031611.lvlib\\设备状态2"(i16 32 ("设备状态")) -> ()  [unwired: 1 in, 1 out]
                      }
                      frame 4 {
                        n562 = shared-variable "我的电脑\\A17031611.lvlib\\设备状态2"(i16 31 ("设备状态")) -> ()  [unwired: 1 in, 1 out]
                      }
                    }
                  }
                  frame 31 {
                    n563 = control-ref of="?"() -> (w411:refnum<vi>)
                    n564 = call "浮动通知2.vi"("通知内容"="请安装固定螺栓1并确认扭矩！" ("Status")) -> ()  [unwired: 11 in]
                    n565 = call "Colour -ECU.vi"("result"="等待", "colourRef"=w411) -> ()  [unwired: 9 in, 1 out]
                  }
                  frame 32 {
                    n566 = flat-sequence {
                      frame #0 {
                        n567 = control-ref of="?"() -> (w413:refnum<vi>)
                        n568 = call "Colour.vi"("result"="OK", "colourRef"=w413) -> ()  [unwired: 9 in, 1 out]
                      }
                      frame #1 {
                        n569 = local read "ECU步骤"() -> (w417:T2)
                        n570 = Increment(x=w417) -> (x+1=w416:T2)
                        n571 = local write "STEP2"("步骤" ("STEP2")) -> ()
                        n572 = local write "ECU步骤"(w416) -> ()
                      }
                    }
                  }
                  frame 33 {
                    n573 = control-ref of="?"() -> (w419:refnum<vi>)
                    n574 = call "浮动通知2.vi"("通知内容"="控制器安装螺栓2拧紧确认！" ("Status")) -> ()  [unwired: 11 in]
                    n575 = call "Colour -ECU.vi"("result"="等待", "colourRef"=w419) -> ()  [unwired: 9 in, 1 out]
                  }
                  frame 34 {
                    n576 = flat-sequence {
                      frame #0 {
                        n577 = control-ref of="?"() -> (w422:refnum<vi>)
                        n578 = call "Colour -ECU.vi"("result"="OK", "colourRef"=w422) -> ()  [unwired: 9 in, 1 out]
                      }
                      frame #1 {
                        n579 = local read "ECU步骤"() -> (w425:T2)
                        n580 = Increment(x=w425) -> (x+1=w424:T2)
                        n581 = local write "STEP2"("步骤" ("STEP2")) -> ()
                        n582 = local write "ECU步骤"(w424) -> ()
                      }
                    }
                  }
                  frame 35 {
                    n583 = control-ref of="请取降噪块1"() -> (w427:refnum<vi>)
                    n584 = call "浮动通知2.vi"("通知内容"="控制器安装螺栓3拧紧确认!") -> ()  [unwired: 11 in]
                    n585 = call "Colour -ECU.vi"("result"="等待", "colourRef"=w427) -> ()  [unwired: 9 in, 1 out]
                  }
                  frame 36 {
                    n586 = flat-sequence {
                      frame #0 {
                        n587 = control-ref of="请取降噪块1"() -> (w430:refnum<vi>)
                        n588 = call "Colour -ECU.vi"("result"="等待", "colourRef"=w430) -> ()  [unwired: 9 in, 1 out]
                      }
                      frame #1 {
                        n589 = local read "ECU步骤"() -> (w433:T2)
                        n590 = local write "STEP2"("步骤" ("STEP2")) -> ()
                        n591 = Increment(x=w433) -> (x+1=w432:T2)
                        n592 = local write "ECU步骤"(w432) -> ()
                      }
                    }
                  }
                  frame 40 {
                  }
                  frame 41 {
                    n593 = control-ref of="请取降噪块2"() -> (w435:refnum<vi>)
                    n594 = call "浮动通知2.vi"("通知内容"="请安装控制器支架1并确认扭矩！" ("Status")) -> ()  [unwired: 11 in]
                    n595 = call "Colour -ECU.vi"("result"="等待", "colourRef"=w435) -> ()  [unwired: 9 in, 1 out]
                  }
                  frame 42 {
                    n596 = flat-sequence {
                      frame #0 {
                        n597 = control-ref of="请取降噪块2"() -> (w438:refnum<vi>)
                        n598 = call "Colour -ECU.vi"("result"="OK", "colourRef"=w438) -> ()  [unwired: 9 in, 1 out]
                      }
                      frame #1 {
                        n599 = local read "ECU步骤"() -> (w441:T2)
                        n600 = Increment(x=w441) -> (x+1=w440:T2)
                        n601 = local write "STEP2"("步骤" ("STEP2")) -> ()
                        n602 = local write "ECU步骤"(w440) -> ()
                      }
                    }
                  }
                  frame 43 {
                    n603 = control-ref of="请取锁紧块"() -> (w443:refnum<vi>)
                    n604 = call "Colour -ECU.vi"("result"="等待", "colourRef"=w443) -> ()  [unwired: 9 in, 1 out]
                    n605 = call "浮动通知2.vi"("通知内容"="请安装控制器支架2并确认扭矩！" ("Status")) -> ()  [unwired: 11 in]
                  }
                  frame 44 {
                    n606 = flat-sequence {
                      frame #0 {
                        n607 = control-ref of="请取锁紧块"() -> (w446:refnum<vi>)
                        n608 = call "Colour -ECU.vi"("result"="OK", "colourRef"=w446) -> ()  [unwired: 9 in, 1 out]
                      }
                      frame #1 {
                        n609 = local read "ECU步骤"() -> (w448:T2)
                        n610 = Increment(x=w448) -> (x+1=w449:T2)
                        n611 = local write "STEP2"("步骤" ("STEP2")) -> ()
                        n612 = local write "ECU步骤"(w449) -> ()
                      }
                    }
                  }
                  frame 45 {
                    n613 = control-ref of="请安装推力滚针轴承"() -> (w451:refnum<vi>)
                    n614 = call "浮动通知2.vi"("通知内容"="请安装控制器支架3并确认扭矩") -> ()  [unwired: 11 in]
                    n615 = call "Colour -ECU.vi"("result"="等待", "colourRef"=w451) -> ()  [unwired: 9 in, 1 out]
                  }
                  frame 46 {
                    n616 = flat-sequence {
                      frame #0 {
                        n617 = control-ref of="请安装推力滚针轴承"() -> (w454:refnum<vi>)
                        n618 = call "Colour -ECU.vi"("result"="OK", "colourRef"=w454) -> ()  [unwired: 9 in, 1 out]
                      }
                      frame #1 {
                        n619 = local read "ECU步骤"() -> (w456:T2)
                        n620 = Increment(x=w456) -> (x+1=w457:T2)
                        n621 = local write "STEP2"("步骤" ("STEP2")) -> ()
                        n622 = local write "ECU步骤"(w457) -> ()
                      }
                    }
                  }
                  frame 47 {
                    n623 = control-ref of="请安装挡片"() -> (w459:refnum<vi>)
                    n624 = call "浮动通知2.vi"("通知内容"="请安装控制器支架3并确认扭矩") -> ()  [unwired: 11 in]
                    n625 = call "Colour -ECU.vi"("result"="等待", "colourRef"=w459) -> ()  [unwired: 9 in, 1 out]
                  }
                  frame 48 {
                    n626 = flat-sequence {
                      frame #0 {
                        n627 = control-ref of="请安装挡片"() -> (w462:refnum<vi>)
                        n628 = call "Colour -ECU.vi"("result"="OK", "colourRef"=w462) -> ()  [unwired: 9 in, 1 out]
                      }
                      frame #1 {
                        n629 = local read "ECU步骤"() -> (w464:T2)
                        n630 = Increment(x=w464) -> (x+1=w465:T2)
                        n631 = local write "STEP2"("步骤" ("STEP2")) -> ()
                        n632 = local write "ECU步骤"(w465) -> ()
                      }
                    }
                  }
                  frame 60 {
                    n633 = Index Array(array=w469, index=4 ("索引")) -> ()  [unwired: 1 out]
                    n634 = call "浮动通知2.vi"("通知内容"="请取记号笔标记!") -> ()  [unwired: 11 in]
                    n635 = control-ref of="请安装锁紧螺母"() -> (w467:refnum<vi>)
                    n636 = call "Colour -ECU.vi"("result"="等待", "colourRef"=w467) -> ()  [unwired: 9 in, 1 out]
                  }
                  frame 61 {
                    n637 = Index Array(array=w471, index #1=4 ("索引")) -> ()  [unwired: 1 in, 2 out]
                    n638 = flat-sequence {
                      frame #0 {
                        n639 = control-ref of="请安装锁紧螺母"() -> (w473:refnum<vi>)
                        n640 = call "Colour.vi"("result"="OK", "colourRef"=w473) -> ()  [unwired: 9 in, 1 out]
                      }
                      frame #1 {
                        n641 = local read "ECU步骤"() -> (w476:T2)
                        n642 = Increment(x=w476) -> (x+1=w477:T2)
                        n643 = local write "STEP2"("步骤" ("STEP2")) -> ()
                        n644 = local write "ECU步骤"(w477) -> ()
                      }
                    }
                  }
                  frame 70 {
                    n645 = control-ref of="请安装弹簧"() -> (w479:refnum<vi>)
                    n646 = call "Colour -ECU.vi"("result"="等待", "colourRef"=w479) -> ()  [unwired: 9 in, 1 out]
                    n647 = call "浮动通知2.vi"("通知内容"="请取轧带！" ("Status")) -> ()  [unwired: 11 in]
                  }
                  frame 71 {
                    n648 = flat-sequence {
                      frame #0 {
                        n649 = control-ref of="请安装弹簧"() -> (w483:refnum<vi>)
                        n650 = call "浮动通知2.vi"("通知内容"="完成！" ("Status")) -> ()  [unwired: 11 in]
                        n651 = call "Colour -ECU.vi"("result"="OK", "colourRef"=w483) -> ()  [unwired: 9 in, 1 out]
                      }
                      frame #1 {
                        n652 = local write "STEP2"("步骤" ("STEP2")) -> ()
                        n653 = local write "ECU步骤"(T2."完成" ("ECU步骤")) -> ()
                      }
                    }
                  }
                  frame 81 {
                    n654 = Index Array(array=w487, index #1=8 ("索引")) -> ()  [unwired: 1 in, 2 out]
                    n655 = call "浮动通知2.vi"("通知内容"="完成!") -> ()  [unwired: 11 in]
                    n656 = shared-variable "我的电脑\\A17031611.lvlib\\设备状态2"(i16 200 ("设备状态")) -> ()  [unwired: 1 in, 1 out]
                  }
                  frame 91 {
                    (unwired) "请安装电机扎带并取走工件！" ("Status")
                    n657 = Index Array(array=w490, index #1=5 ("索引")) -> (element #1=w492:refnum<vi>, element #2=w491:refnum<vi>)  [unwired: 1 in]
                    n658 = call "Colour.vi"("result"="OK", "colourRef"=w492) -> ()  [unwired: 9 in, 1 out]
                    n659 = call "Colour.vi"("result"="等待", "colourRef"=w491) -> ()  [unwired: 9 in, 1 out]
                    n660 = shared-variable "我的电脑\\A17031611.lvlib\\设备状态3"(i16 100 ("设备状态")) -> ()  [unwired: 1 in, 1 out]
                  }
                  frame 101 {
                    (unwired) "完成！" ("Status")
                    n661 = Index Array(array=w497, index #1=6 ("索引")) -> (element #1=w499:refnum<vi>, element #2=w498:refnum<vi>)  [unwired: 1 in]
                    n662 = call "Colour.vi"("result"="OK", "colourRef"=w499) -> ()  [unwired: 9 in, 1 out]
                    n663 = call "Colour.vi"("result"="等待", "colourRef"=w498) -> ()  [unwired: 9 in, 1 out]
                    n664 = shared-variable "我的电脑\\A17031611.lvlib\\设备状态3"(i16 110 ("设备状态")) -> ()  [unwired: 1 in, 1 out]
                  }
                  frame 200 {
                    n665 = global read "Global.vi" "检测结果"() -> (w513:refnum<vi>)
                    n666 = global write "Global1.vi" "ECU工位生产结果"("OK" ("电机工位生产结果")) -> ()
                    n667 = call "浮动通知2.vi"("通知内容"="产品合格！" ("Status")) -> ()  [unwired: 11 in]
                    n668 = call "Colour.vi"("result"="OK", "colourRef"=w513) -> ()  [unwired: 9 in, 1 out]
                    n669 = global read "Global.vi" "ECU结果显示"() -> (w511:refnum<vi>)
                    n670 = property class="Str"(reference=w511, "Value"="OK" ("结果显示")) -> (reference out=w508:refnum<vi>)  [unwired: 1 in, 1 out]
                    n671 = global read "Global1.vi" "联机模式"() -> (w505:enum16{"单机", "追溯"})
                    n672 = property class="Str"(reference=w508, "Text.TextColor"=u32 9567230) -> ()  [unwired: 1 in, 2 out]
                    n673 = case shown="\"追溯\"" w505 {
                      tunnel: ["自动" "录入数据库" ("STEP3")] -> w504
                      frame "单机", Default {
                        n674 = shared-variable "我的电脑\\A17031611.lvlib\\设备状态2"(i16 6 ("设备状态")) -> ()  [unwired: 1 in, 1 out]
                        n675 = local write "ECU步骤"(T2."控制器安装螺栓1" ("ECU步骤")) -> ()
                      }
                      frame "追溯" {
                      }
                    }
                    n676 = local write "STEP2"(w504) -> ()
                  }
                  frame 201 {
                    (unwired) "产品不合格！" ("Status")
                    n677 = global read "Global.vi" "检测结果"() -> (w522:refnum<vi>)
                    n678 = call "Colour.vi"("result"="NG", "colourRef"=w522) -> ()  [unwired: 9 in, 1 out]
                    n679 = global read "Global.vi" "电机结果显示"() -> (w521)
                    n680 = property class="Str"(reference=w521, "Value"="NG" ("结果显示")) -> (reference out=w520:refnum<vi>)  [unwired: 1 in, 1 out]
                    n681 = property class="Str"(reference=w520, "Text.TextColor"=u32 16711680) -> ()  [unwired: 1 in, 2 out]
                  }
                  frame 999 {
                    n682 = for {
                      tunnel: w524 -> [w527] mode=indexing
                      n683 = call "Colour.vi"("result"="", "colourRef"=w527) -> ()  [unwired: 9 in, 1 out]
                    }
                    n684 = call "浮动通知2.vi"("通知内容"="请重新安装固定螺栓！" ("Status")) -> ()  [unwired: 11 in]
                    n685 = shared-variable "我的电脑\\A17031611.lvlib\\设备状态2"(i16 31 ("设备状态")) -> ()  [unwired: 1 in, 1 out]
                  }
                  frame 1024 {
                    n686 = global read "Global.vi" "ECU自动"() -> (w530:refnum<vi>)
                    n687 = property class="Bool (严格)"(reference=w530, "Value"=FALSE) -> ()  [unwired: 1 in, 2 out]
                  }
                  frame 3721 {
                    (unwired) "产品不合格程序锁定！" ("Status")
                    n688 = local write "STEP3"("不合格锁定" ("STEP")) -> ()
                  }
                  frame 3722 {
                    n689 = global read "Global.vi" "ECU自动"() -> (w533:refnum<vi>)
                    n690 = property class="Bool (严格)"(reference=w533, "Value"=FALSE) -> ()  [unwired: 1 in, 2 out]
                  }
                  frame 3723 {
                    (unwired) "请取出不合格产品并摆放至不合格品区！" ("Status")
                  }
                }
              }
              frame "录入数据库" {
                n691 = stacked-sequence {
                  frame #0 {
                    n692 = Get Date/Time String(date format (0)=enum16{"short", "long", "abbreviated"}."short" ("日期格式(0)"), want seconds? (F)=FALSE ("需要秒？(F)")) -> (date string=w543:string, time string=w544:string)  [unwired: 1 in]
                    n693 = global read "Global1.vi" "DEVICE_ID_ECU"() -> (w547:string)
                    n694 = global read "Global1.vi" "CODE_ID_ECU"() -> (w546:string)
                    n695 = global read "Global1.vi" "ECU工位生产结果"() -> (w538:string)
                    n696 = global read "Global1.vi" "USER_ID"() -> (w545:string)
                    n697 = Concatenate Strings(w543, " " ("字符串"), w544) -> (w539:string)
                    n698 = Decimal String To Number(string=w547, default (0L)=i64 0 ("默认(0 I32)")) -> (number=w536:i64)  [unwired: 1 in, 1 out]
                    n699 = Decimal String To Number(string=w545, default (0L)=i64 0 ("默认(0 I32)")) -> (number=w535:i64)  [unwired: 1 in, 1 out]
                    n700 = Decimal String To Number(string=w546, default (0L)=i64 0 ("默认(0 I32)")) -> (number=w534:i64)  [unwired: 1 in, 1 out]
                    n701 = global read "Global1.vi" "联机模式"() -> (w554:enum16{"单机", "追溯"})
                    n702 = Search and Replace String(replace all?=TRUE ("替换全部？(F)"), input string=w539, search string="/" ("替换字符串(\"\")"), replace string="-" ("替换字符串(\"\")")) -> (result string=w537:string)  [unwired: 4 in, 3 out]
                    n703 = Bundle(w536, w535, w534, "ECU工位生产结果"=w538, "result string"=w537) -> (w560:T7)  [unwired: 1 in]
                    n704 = call "GetSQLstring.vi"("联机模式"=w554) -> ("错误输出"=w557:errorcluster, "连接字符串"=w556:string)  [unwired: 9 in]
                    n705 = Build Array(w560) -> (w561:T8)
                    n706 = call-poly <vilib>:"DB Tools Open Connection.vi"("error in (no error)"=w557, "connection information"=w556) -> ("error out"=w555:errorcluster, "connection reference"=w558:T6)  [unwired: 6 in]
                    n707 = for {
                      tunnel: w561 -> [w566] mode=indexing
                      tunnel: w558 -> [w564]
                      shift-right: [w562] -> w559
                      shift-left: w555 -> [w569]
                      w565 = string[] ["DEVICE_ID", "USER_ID", "CODE_ID", "RESULT_VALUE", "RESULT_TIME"] ("columns")
                      w567 = "Result" ("table")
                      n708 = call <vilib>:"DB Tools Insert Data.vi"("data"=w566, "error in (no error)"=w569, "columns"=w565, "table"=w567, "connection reference"=w564) -> ("error out"=w568:errorcluster, "connection reference out"=w563:T6)  [unwired: 5 in]
                      n709 = case shown="错误" w568 {
                        selector: w568 -> [w570 w591]
                        tunnel: w565 -> [_ w588]
                        tunnel: w563 -> [w571 w580]
                        tunnel: w567 -> [_ w592]
                        tunnel: w566 -> [_ w584]
                        tunnel: [w571 w579] -> _
                        tunnel: [w570 w578] -> w562
                        frame No Error {
                        }
                        frame Error {
                          n710 = Array Subset(array=w588, index=3 ("长度"), length=2 ("长度")) -> (w589:string[])
                          n711 = Unbundle(w584) -> (w573:i64, w576:i64, "ECU工位生产结果"=w583:string, "result string"=w582:string)  [unwired: 1 out]
                          n712 = Number To Decimal String(number=w576) -> (decimal integer string=w577:string)  [unwired: 1 in]
                          n713 = Number To Decimal String(number=w573) -> (decimal integer string=w572:string)  [unwired: 1 in]
                          n714 = Concatenate Strings("WHERE CODE_ID =" ("condition"), w577, "AND DEVICE_ID = ", w572) -> (w585:string)
                          n715 = Bundle("ECU工位生产结果"=w583, "result string"=w582) -> (w581:T9)  [unwired: 1 in]
                          n716 = call <vilib>:"Clear Errors.vi"("error in (no error)"=w591) -> ("error out"=w590:errorcluster)  [unwired: 5 in, 1 out]
                          n717 = call <vilib>:"DB Tools Update Data.vi"("condition"=w585, "data"=w581, "error in (no error)"=w590, "columns"=w589, "table"=w592, "connection reference"=w580) -> ("error out"=w578:errorcluster, "connection reference out"=w579:T6)  [unwired: 4 in]
                        }
                      }
                    }
                    n718 = call <vilib>:"Simple Error Handler.vi"("error in (no error)"=w559) -> ()  [unwired: 4 in, 5 out]
                  }
                  frame #1 {
                    n719 = global read "Global1.vi" "CODE_ID_ECU"() -> (w594:string)
                    n720 = global read "Global1.vi" "控制器码"() -> (w593:string)
                    n721 = Format Into String(format string="UPDATE\ndbo.[Code]\nSET dbo.[Code].CODE_ECU = '%s'\n\nWHERE\ndbo.[Code].CODE_ID = %s\n" ("格式字符串"), w593, w594) -> (resulting string=w597:string)  [unwired: 2 in, 1 out]
                    n722 = call "SQL_query.vi"("SQL query"=w597, "联机模式"=enum16{"单机", "联网"}."联网") -> ()  [unwired: 1 in, 3 out]
                  }
                  frame #2 {
                  }
                  frame #3 {
                    n723 = call "浮动通知2.vi"("通知内容"="ECU工位数据录入成功！" ("Status")) -> ()  [unwired: 11 in]
                    n724 = local write "STEP2"("等待" ("STEP2")) -> ()
                    n725 = shared-variable "我的电脑\\A17031611.lvlib\\设备状态2"(i16 6 ("设备状态")) -> ()  [unwired: 1 in, 1 out]
                  }
                }
              }
              frame "步骤" {
                n726 = case shown="\"控制器安装螺栓1\", 默认" "ECU步骤" {
                  selector: "ECU步骤" -> [w604 _]
                  tunnel: [w603 "等待"] -> w601
                  frame "控制器安装螺栓1", Default {
                    n727 = global read "Global.vi" "手柄安装步骤"() -> (w606:bool[])
                    n728 = Index Array(array=w606, index=w604) -> (element=w605:bool)
                    n729 = case shown="真" w605 {
                      tunnel: w604 -> [_ w611]
                      tunnel: ["步骤" w610] -> w603
                      frame False {
                        n730 = local read "ECU步骤"() -> (w609:T2)
                        n731 = Increment(x=w609) -> (x+1=w608:T2)
                        n732 = local write "ECU步骤"(w608) -> ()
                      }
                      frame True {
                        n733 = case shown="\"安装线卡轧带\"" w611 {
                          tunnel: ["等待" "等待" "等待" "等待" "等待" "等待" "等待" "等待" "等待"] -> w610
                          frame "控制器安装螺栓1", Default {
                            n734 = shared-variable "我的电脑\\A17031611.lvlib\\设备状态2"(i16 31 ("设备状态控制字")) -> ()  [unwired: 1 in, 1 out]
                          }
                          frame "控制器安装螺栓2" {
                            n735 = shared-variable "我的电脑\\A17031611.lvlib\\设备状态2"(i16 33 ("设备状态控制字")) -> ()  [unwired: 1 in, 1 out]
                          }
                          frame "控制器安装螺栓3" {
                            n736 = shared-variable "我的电脑\\A17031611.lvlib\\设备状态2"(i16 35 ("设备状态控制字")) -> ()  [unwired: 1 in, 1 out]
                          }
                          frame "安装支架螺栓1" {
                            n737 = shared-variable "我的电脑\\A17031611.lvlib\\设备状态2"(i16 41 ("设备状态控制字")) -> ()  [unwired: 1 in, 1 out]
                          }
                          frame "安装支架螺栓2" {
                            n738 = shared-variable "我的电脑\\A17031611.lvlib\\设备状态2"(i16 43 ("设备状态控制字")) -> ()  [unwired: 1 in, 1 out]
                          }
                          frame "安装支架螺栓3" {
                            n739 = shared-variable "我的电脑\\A17031611.lvlib\\设备状态2"(i16 45 ("设备状态控制字")) -> ()  [unwired: 1 in, 1 out]
                          }
                          frame "安装支架螺栓4" {
                            n740 = shared-variable "我的电脑\\A17031611.lvlib\\设备状态2"(i16 47 ("设备状态控制字")) -> ()  [unwired: 1 in, 1 out]
                          }
                          frame "涂色标" {
                            n741 = shared-variable "我的电脑\\A17031611.lvlib\\设备状态2"(i16 60 ("设备状态控制字")) -> ()  [unwired: 1 in, 1 out]
                          }
                          frame "安装线卡轧带" {
                            n742 = shared-variable "我的电脑\\A17031611.lvlib\\设备状态2"(i16 70 ("设备状态控制字")) -> ()  [unwired: 1 in, 1 out]
                          }
                        }
                      }
                    }
                  }
                  frame "完成" {
                    n743 = shared-variable "我的电脑\\A17031611.lvlib\\设备状态2"(i16 81 ("设备状态控制字")) -> ()  [unwired: 1 in, 1 out]
                  }
                }
                n744 = local write "STEP2"(w601) -> ()
              }
            }
            n745 = case shown="\"初始化\"" "STEP1" {
              frame "等待", Default {
                n746 = local write "STEP1"("自动" ("STEP1")) -> ()
                n747 = Wait (ms)(milliseconds to wait=u32 200 ("等待时间（毫秒）")) -> ()  [unwired: 1 out]
              }
              frame "初始化" {
                n748 = local write "STEP1"("步骤" ("STEP")) -> ()
                n749 = local write "控制器支架"(T1."控制器支架螺栓1" ("控制器支架")) -> ()
              }
              frame "自动" {
                # "5=31\n4=32\n3=33\n2=34\n1=35"
                n750 = shared-variable "我的电脑\\A17031611.lvlib\\控制器支架螺栓数量"() -> (w58:i16)  [unwired: 1 in, 1 out]
                n751 = shared-variable "我的电脑\\A17031611.lvlib\\设备状态1"() -> (w59:i16)  [unwired: 1 in, 1 out]
                n752 = global read "A170316-11.vi" "控制器支架LED"() -> (w60:refnum<vi>[])
                n753 = case shown="10" w59 {
                  tunnel: w60 -> [_ _ _ _ _ _ _ _ _ _ _ _ _ w105 _ w115 w122 w138]
                  tunnel: w58 -> [_ _ _ _ _ _ _ _ _ _ _ _ _ _ _ _ _ _]
                  frame 0, Default {
                  }
                  frame 10 {
                    n754 = local write "STEP1"("初始化" ("STEP1")) -> ()
                  }
                  frame 30 {
                    n755 = control-ref of="控制器支架螺栓1拧紧确认"() -> (w63:refnum<vi>)
                    n756 = call "Colour.vi"("result"="等待", "colourRef"=w63) -> ()  [unwired: 9 in, 1 out]
                    n757 = call "浮动通知2.vi"("通知内容"="请安装第一颗螺丝并拧紧！" ("Status")) -> ()  [unwired: 11 in]
                  }
                  frame 31 {
                    n758 = flat-sequence {
                      frame #0 {
                        n759 = control-ref of="控制器支架螺栓1拧紧确认"() -> (w66:refnum<vi>)
                        n760 = call "Colour.vi"("result"="OK", "colourRef"=w66) -> ()  [unwired: 9 in, 1 out]
                      }
                      frame #1 {
                        n761 = local read "控制器支架"() -> (w69:T1)
                        n762 = Increment(x=w69) -> (x+1=w68:T1)
                        n763 = local write "STEP1"("步骤" ("STEP1")) -> ()
                        n764 = local write "控制器支架"(w68) -> ()
                      }
                    }
                  }
                  frame 32 {
                    n765 = control-ref of="控制器支架螺栓2拧紧确认"() -> (w71:refnum<vi>)
                    n766 = call "Colour.vi"("result"="等待", "colourRef"=w71) -> ()  [unwired: 9 in, 1 out]
                    n767 = call "浮动通知2.vi"("通知内容"="请安装第二颗螺丝并拧紧！" ("Status")) -> ()  [unwired: 11 in]
                  }
                  frame 33 {
                    n768 = flat-sequence {
                      frame #0 {
                        n769 = control-ref of="控制器支架螺栓2拧紧确认"() -> (w73:refnum<vi>)
                        n770 = call "Colour.vi"("result"="OK", "colourRef"=w73) -> ()  [unwired: 9 in, 1 out]
                      }
                      frame #1 {
                        n771 = local read "控制器支架"() -> (w76:T1)
                        n772 = Increment(x=w76) -> (x+1=w75:T1)
                        n773 = local write "控制器支架"(w75) -> ()
                        n774 = local write "STEP1"("步骤" ("STEP1")) -> ()
                      }
                    }
                  }
                  frame 34 {
                    # "控制器支架螺栓1"
                    n775 = control-ref of="控制器支架螺栓3拧紧确认"() -> (w78:refnum<vi>)
                    n776 = call "Colour.vi"("result"="等待", "colourRef"=w78) -> ()  [unwired: 9 in, 1 out]
                    n777 = call "浮动通知2.vi"("通知内容"="请安装第三颗螺丝并拧紧！" ("Status")) -> ()  [unwired: 11 in]
                  }
                  frame 35 {
                    n778 = flat-sequence {
                      frame #0 {
                        n779 = control-ref of="控制器支架螺栓3拧紧确认"() -> (w81:refnum<vi>)
                        n780 = call "Colour.vi"("result"="OK", "colourRef"=w81) -> ()  [unwired: 9 in, 1 out]
                      }
                      frame #1 {
                        n781 = local read "控制器支架"() -> (w84:T1)
                        n782 = Increment(x=w84) -> (x+1=w83:T1)
                        n783 = local write "控制器支架"(w83) -> ()
                        n784 = local write "STEP1"("步骤" ("STEP1")) -> ()
                      }
                    }
                  }
                  frame 36 {
                    n785 = control-ref of="控制器支架螺栓4拧紧确认"() -> (w86:refnum<vi>)
                    n786 = call "浮动通知2.vi"("通知内容"="请安装第四颗螺丝并拧紧！" ("Status")) -> ()  [unwired: 11 in]
                    n787 = call "Colour.vi"("result"="等待", "colourRef"=w86) -> ()  [unwired: 9 in, 1 out]
                  }
                  frame 37 {
                    n788 = flat-sequence {
                      frame #0 {
                        n789 = control-ref of="控制器支架螺栓4拧紧确认"() -> (w89:refnum<vi>)
                        n790 = call "Colour.vi"("result"="OK", "colourRef"=w89) -> ()  [unwired: 9 in, 1 out]
                      }
                      frame #1 {
                        n791 = local read "控制器支架"() -> (w92:T1)
                        n792 = Increment(x=w92) -> (x+1=w91:T1)
                        n793 = local write "控制器支架"(w91) -> ()
                        n794 = local write "STEP1"("步骤" ("STEP1")) -> ()
                      }
                    }
                  }
                  frame 38 {
                    n795 = control-ref of="控制器支架螺栓5拧紧确认"() -> (w94:refnum<vi>)
                    n796 = call "Colour.vi"("result"="等待", "colourRef"=w94) -> ()  [unwired: 9 in, 1 out]
                    n797 = call "浮动通知2.vi"("通知内容"="请安装第五颗螺丝并拧紧！" ("Status")) -> ()  [unwired: 11 in]
                  }
                  frame 39 {
                    n798 = flat-sequence {
                      frame #0 {
                        n799 = control-ref of="控制器支架螺栓5拧紧确认"() -> (w97:refnum<vi>)
                        n800 = call "Colour.vi"("result"="OK", "colourRef"=w97) -> ()  [unwired: 9 in, 1 out]
                      }
                      frame #1 {
                        n801 = local read "控制器支架"() -> (w100:T1)
                        n802 = Increment(x=w100) -> (x+1=w99:T1)
                        n803 = local write "控制器支架"(w99) -> ()
                        n804 = local write "STEP1"("步骤" ("STEP1")) -> ()
                      }
                    }
                  }
                  frame 60 {
                    n805 = control-ref of="控制器支架涂色标"() -> (w102:refnum<vi>)
                    n806 = call "Colour.vi"("result"="等待", "colourRef"=w102) -> ()  [unwired: 9 in, 1 out]
                    n807 = call "浮动通知2.vi"("通知内容"="请控制器固定螺栓涂色标！" ("Status")) -> ()  [unwired: 11 in]
                  }
                  frame 61 {
                    n808 = Index Array(array=w105, index #1=4 ("索引")) -> ()  [unwired: 1 in, 2 out]
                    n809 = flat-sequence {
                      frame #0 {
                        n810 = control-ref of="控制器支架涂色标"() -> (w108:refnum<vi>)
                        n811 = call "Colour.vi"("result"="OK", "colourRef"=w108) -> ()  [unwired: 9 in, 1 out]
                      }
                      frame #1 {
                        n812 = local read "控制器支架"() -> (w111:T1)
                        n813 = Increment(x=w111) -> (x+1=w110:T1)
                        n814 = local write "控制器支架"(w110) -> ()
                        n815 = local write "STEP1"("步骤" ("STEP1")) -> ()
                      }
                    }
                  }
                  frame 70 {
                    n816 = control-ref of="控制器支架安装线卡扎带"() -> (w112:refnum<vi>)
                    n817 = call "Colour.vi"("result"="等待", "colourRef"=w112) -> ()  [unwired: 9 in, 1 out]
                    n818 = call "浮动通知2.vi"("通知内容"="请安装轧带并取走工件！" ("Status")) -> ()  [unwired: 11 in]
                  }
                  frame 81 {
                    n819 = Index Array(array=w115, index=6 ("索引")) -> ()  [unwired: 1 out]
                    n820 = flat-sequence {
                      frame #0 {
                        n821 = control-ref of="控制器支架安装线卡扎带"() -> (w118:refnum<vi>)
                        n822 = call "Colour.vi"("result"="OK", "colourRef"=w118) -> ()  [unwired: 9 in, 1 out]
                      }
                      frame #1 {
                        n823 = local read "控制器支架"() -> (w121:T1)
                        n824 = Increment(x=w121) -> (x+1=w120:T1)
                        n825 = local write "控制器支架"(w120) -> ()
                        n826 = local write "STEP1"("步骤" ("STEP1")) -> ()
                      }
                    }
                  }
                  frame 91 {
                    n827 = for {
                      tunnel: w122 -> [w126] mode=indexing
                      n828 = call "Colour.vi"("result"="", "colourRef"=w126) -> ()  [unwired: 9 in, 1 out]
                    }
                    n829 = shared-variable "我的电脑\\A17031611.lvlib\\设备状态1"(i16 10 ("设备状态")) -> ()  [unwired: 1 in, 1 out]
                    n830 = local write "STEP1"("初始化" ("STEP1")) -> ()
                    n831 = call "浮动通知2.vi"("通知内容"="控制器和支架合装完成！" ("Status")) -> ()  [unwired: 11 in]
                  }
                  frame 999 {
                    n832 = Index Array(array=w138, index #1=0 ("索引")) -> (element #1=w141:refnum<vi>, element #2=w135:refnum<vi>, element #3=w133:refnum<vi>, element #4=w131:refnum<vi>, element #5=w128:refnum<vi>)  [unwired: 4 in]
                    n833 = call "Colour.vi"("result"="", "colourRef"=w128) -> ()  [unwired: 9 in, 1 out]
                    n834 = call "Colour.vi"("result"="", "colourRef"=w135) -> ()  [unwired: 9 in, 1 out]
                    n835 = call "Colour.vi"("result"="", "colourRef"=w133) -> ()  [unwired: 9 in, 1 out]
                    n836 = call "Colour.vi"("result"="", "colourRef"=w131) -> ()  [unwired: 9 in, 1 out]
                    n837 = call "Colour.vi"("result"="NG", "colourRef"=w141) -> ()  [unwired: 9 in, 1 out]
                    n838 = call "浮动通知2.vi"("通知内容"="安装固定螺栓未完成，请重新安装！" ("Status")) -> ()  [unwired: 11 in]
                    n839 = shared-variable "我的电脑\\A17031611.lvlib\\设备状态1"(i16 10 ("设备状态")) -> ()  [unwired: 1 in, 1 out]
                  }
                }
              }
              frame "步骤" {
                n840 = case shown="\"控制器支架螺栓1\", 默认" "控制器支架" {
                  selector: "控制器支架" -> [w145 _]
                  tunnel: [w144 "自动"] -> w142
                  frame "控制器支架螺栓1", Default {
                    n841 = global read "Global.vi" "控制器支架"() -> (w147:bool[])
                    n842 = Index Array(array=w147, index=w145) -> (element=w146:bool)
                    n843 = case shown="真" w146 {
                      tunnel: w145 -> [_ w152]
                      tunnel: ["步骤" w151] -> w144
                      frame False {
                        n844 = local read "控制器支架"() -> (w150:T1)
                        n845 = Increment(x=w150) -> (x+1=w149:T1)
                        n846 = local write "控制器支架"(w149) -> ()
                      }
                      frame True {
                        n847 = case shown="\"安装线卡轧带\"" w152 {
                          tunnel: ["等待" "等待" "等待" "等待" "等待" "等待" "等待"] -> w151
                          frame "控制器支架螺栓1", Default {
                            n848 = shared-variable "我的电脑\\A17031611.lvlib\\设备状态1"(i16 30 ("设备状态1")) -> ()  [unwired: 1 in, 1 out]
                          }
                          frame "控制器支架螺栓2" {
                            n849 = shared-variable "我的电脑\\A17031611.lvlib\\设备状态1"(i16 32 ("设备状态1")) -> ()  [unwired: 1 in, 1 out]
                          }
                          frame "控制器支架螺栓3" {
                            n850 = shared-variable "我的电脑\\A17031611.lvlib\\设备状态1"(i16 34 ("设备状态1")) -> ()  [unwired: 1 in, 1 out]
                          }
                          frame "控制器支架螺栓4" {
                            n851 = shared-variable "我的电脑\\A17031611.lvlib\\设备状态1"(i16 36 ("设备状态1")) -> ()  [unwired: 1 in, 1 out]
                          }
                          frame "控制器支架螺栓5" {
                            n852 = shared-variable "我的电脑\\A17031611.lvlib\\设备状态1"(i16 38 ("设备状态1")) -> ()  [unwired: 1 in, 1 out]
                          }
                          frame "涂色标" {
                            n853 = shared-variable "我的电脑\\A17031611.lvlib\\设备状态1"(i16 60 ("设备状态1")) -> ()  [unwired: 1 in, 1 out]
                          }
                          frame "安装线卡轧带" {
                            n854 = shared-variable "我的电脑\\A17031611.lvlib\\设备状态1"(i16 70 ("设备状态1")) -> ()  [unwired: 1 in, 1 out]
                          }
                        }
                      }
                    }
                  }
                  frame "完成" {
                    n855 = shared-variable "我的电脑\\A17031611.lvlib\\设备状态1"(i16 91 ("设备状态")) -> ()  [unwired: 1 in, 1 out]
                  }
                }
                n856 = local write "STEP1"(w142) -> ()
              }
            }
            n857 = global read "Global.vi" "程序关闭"() -> (w53:bool)
          }
        }
        frame Enabled {
        }
      }
      n858 = while {
        stop <- w1108 stop-if-true
        n859 = global read "Global.vi" "产品型号"() -> (w1109:string)
        n860 = Wait Until Next ms Multiple(millisecond multiple=u32 5 ("毫秒倍数")) -> ()  [unwired: 1 out]
        n861 = call "Is Value Changed.vim"("value"=w1109) -> ("changed or first call?"=w1110:bool)
        n862 = event shown="[1] \"前序OK？\": 值改变" {
          selector: _ -> [_ _ _ _]
          dyn-events: _ -> [_ _ _ _]
          timeout: 5 -> [_ _ _ _]
          tunnel: w1109 -> [_ w1129 w1417 _]
          event Timeout {
            w1113 = u16 0
            n863 = event-data() -> ()  [unwired: 1 in, 3 out]
            n864 = feedback #1() -> (w1123:u16)  [unwired: 1 in]
            n865 = feedback-in #1(w1113) -> ()
            n866 = Greater Or Equal?(x=w1113, y=i16 5000) -> (x >= y?=w1121:bool)
            n867 = Less?(x=w1113, y=i16 5200) -> (x < y?=w1122:bool)
            n868 = Equal?(x=w1113, y=w1123) -> (x = y?=w1120:bool)
            n869 = global read "Global.vi" "报警图标"() -> (w1115:refnum<vi>)
            n870 = And(x=w1121, y=w1122) -> (x .and. y?=w1114:bool)
            n871 = property class="Bool"(reference=w1115, "Value"=w1114) -> ()  [unwired: 1 in, 2 out]
            n872 = Bundle By Name(cluster=errorcluster {"status"=FALSE, "code"=0, "source"=""} ("错误常量"), "status"=w1114, "code"=w1113) -> (w1119:errorcluster)
            n873 = case shown="真" w1120 {
              tunnel: w1119 -> [w1128 _]
              frame False {
                n874 = call "报警处理.vi"("错误常量"=w1128) -> ()  [unwired: 9 in, 2 out]
              }
              frame True {
              }
            }
            n875 = case shown="0" w1113 {
              frame 0 {
                n876 = global read "Global.vi" "报警图标"() -> (w1124:refnum<vi>)
                n877 = property class="Bool"(reference=w1124, "Visible"=FALSE ("可见")) -> ()  [unwired: 1 in, 2 out]
              }
              frame 1, Default {
                n878 = global read "Global.vi" "报警图标"() -> (w1127:refnum<vi>)
                n879 = property class="Bool"(reference=w1127, "Visible"=TRUE ("可见")) -> ()  [unwired: 1 in, 2 out]
              }
            }
          }
          event "前序OK？": Value Change {
            n880 = event-data() -> ()  [unwired: 1 in, 6 out]
            n881 = stacked-sequence {
              tunnel: w1129 -> [_ w1183]
              frame #0 {
                n882 = disable-structure shown="禁用" {
                  frame Disabled {
                    n883 = control-ref of="安装扎带并取走工件"() -> (w1136:refnum<vi>)
                    n884 = control-ref of="请拍照确认"() -> (w1135:refnum<vi>)
                    n885 = control-ref of="?"() -> (w1156:refnum<vi>)
                    n886 = control-ref of="?"() -> (w1153:refnum<vi>)
                    n887 = control-ref of="请安装锁紧螺母"() -> (w1155:refnum<vi>)
                    n888 = control-ref of="安装支架扎带安装"() -> (w1139:refnum<vi>)
                    n889 = control-ref of="请安装弹簧"() -> (w1138:refnum<vi>)
                    n890 = control-ref of="请取降噪块1"() -> (w1134:refnum<vi>)
                    n891 = control-ref of="请取降噪块2"() -> (w1158:refnum<vi>)
                    n892 = control-ref of="请安装挡片"() -> (w1130:refnum<vi>)
                    n893 = control-ref of="安装弹性垫圈弹簧并按启动拍照"() -> (w1145:refnum<vi>)
                    n894 = control-ref of="安装扎带并取走工件"() -> (w1140:refnum<vi>)
                    n895 = control-ref of="电机安装螺栓2扭矩确认"() -> (w1143:refnum<vi>)
                    n896 = control-ref of="请安装推力滚针轴承"() -> (w1133:refnum<vi>)
                    n897 = control-ref of="请取锁紧块"() -> (w1157:refnum<vi>)
                    n898 = control-ref of="电机安装螺栓3扭矩确认"() -> (w1131:refnum<vi>)
                    n899 = control-ref of="按启动按钮拍照确认"() -> (w1142:refnum<vi>)
                    n900 = control-ref of="电机安装螺栓1扭矩确认"() -> (w1144:refnum<vi>)
                    n901 = control-ref of="控制器支架涂色标"() -> (w1147:refnum<vi>)
                    n902 = control-ref of="涂色标"() -> (w1141:refnum<vi>)
                    n903 = Build Array(w1158, w1157, w1156, w1153, w1155, w1139, w1138, w1134, w1133, w1130) -> (w1154:refnum<vi>[])
                    n904 = control-ref of="控制器支架螺栓1拧紧确认"() -> (w1151:refnum<vi>)
                    n905 = control-ref of="控制器支架螺栓3拧紧确认"() -> (w1149:refnum<vi>)
                    n906 = for {
                      tunnel: w1154 -> [w1182] mode=indexing
                      i -> [w1181]
                      n907 = Multiply(x=60, y=w1181) -> (x*y=w1176:i32)
                      n908 = Add(x=340 ("y"), y=w1176) -> (x+y=w1178:i32)
                      n909 = Bundle("y"=-500, w1178) -> (w1177:cluster{"y":i32, i32})  [unwired: 1 in]
                      n910 = property class="Bool (严格)"(reference=w1182, "Position"=w1177) -> ()  [unwired: 1 in, 2 out]
                    }
                    n911 = control-ref of="控制器支架安装线卡扎带"() -> (w1137:refnum<vi>)
                    n912 = control-ref of="控制器支架螺栓4拧紧确认"() -> (w1148:refnum<vi>)
                    n913 = Build Array(w1145, w1144, w1143, w1142, w1141, w1140, w1136, w1135, w1131) -> (w1146:refnum<vi>[])
                    n914 = control-ref of="控制器支架螺栓2拧紧确认"() -> (w1150:refnum<vi>)
                    n915 = control-ref of="控制器支架螺栓5拧紧确认"() -> (w1132:refnum<vi>)
                    n916 = for {
                      tunnel: w1146 -> [w1166] mode=indexing
                      i -> [w1165]
                      n917 = Multiply(x=60, y=w1165) -> (x*y=w1163:i32)
                      n918 = Add(x=w1163, y=340) -> (x+y=w1160:i32)
                      n919 = Bundle("y"=-1500, w1160) -> (w1159:cluster{"y":i32, i32})  [unwired: 1 in]
                      n920 = property class="Bool (严格)"(reference=w1166, "Position"=w1159) -> ()  [unwired: 1 in, 2 out]
                    }
                    n921 = Build Array(w1151, w1150, w1149, w1148, w1147, w1137, w1132) -> (w1152:refnum<vi>[])
                    n922 = for {
                      tunnel: w1152 -> [w1174] mode=indexing
                      i -> [w1173]
                      n923 = Multiply(x=60, y=w1173) -> (x*y=w1171:i32)
                      n924 = Add(x=w1171, y=345) -> (x+y=w1168:i32)
                      n925 = Bundle("y"=-1000, w1168) -> (w1167:cluster{"y":i32, i32})  [unwired: 1 in]
                      n926 = property class="Bool (严格)"(reference=w1174, "Position"=w1167) -> ()  [unwired: 1 in, 2 out]
                    }
                  }
                  frame Enabled {
                  }
                }
              }
              frame #1 {
                n927 = disable-structure shown="禁用" {
                  disable-tunnel: w1183 -> [w1184 _]
                  frame Disabled {
                    n928 = case shown="\"R128\"" w1184 {
                      frame Default {
                      }
                      frame "R92A" {
                        n929 = control-ref of="?"() -> (w1189:refnum<vi>)
                        n930 = control-ref of="请安装挡片"() -> (w1191:refnum<vi>)
                        n931 = control-ref of="?"() -> (w1190:refnum<vi>)
                        n932 = control-ref of="请取降噪块2"() -> (w1194:refnum<vi>)
                        n933 = control-ref of="请安装推力滚针轴承"() -> (w1192:refnum<vi>)
                        n934 = control-ref of="请取降噪块1"() -> (w1188:refnum<vi>)
                        n935 = control-ref of="请安装锁紧螺母"() -> (w1187:refnum<vi>)
                        n936 = control-ref of="请取锁紧块"() -> (w1193:refnum<vi>)
                        n937 = control-ref of="安装弹性垫圈弹簧并按启动拍照"() -> (w1201:refnum<vi>)
                        n938 = control-ref of="电机安装螺栓3扭矩确认"() -> (w1195:refnum<vi>)
                        n939 = control-ref of="电机安装螺栓1扭矩确认"() -> (w1200:refnum<vi>)
                        n940 = control-ref of="电机安装螺栓2扭矩确认"() -> (w1199:refnum<vi>)
                        n941 = control-ref of="按启动按钮拍照确认"() -> (w1198:refnum<vi>)
                        n942 = control-ref of="安装扎带并取走工件"() -> (w1196:refnum<vi>)
                        n943 = Build Array(w1194, w1193, w1192, w1191, w1190, w1189, w1188, w1187) -> (w1186:refnum<vi>[])
                        n944 = control-ref of="涂色标"() -> (w1197:refnum<vi>)
                        n945 = for {
                          tunnel: w1186 -> [w1231] mode=indexing
                          i -> [w1230]
                          n946 = Multiply(x=60, y=w1230) -> (x*y=w1225:i32)
                          n947 = Add(x=340 ("y"), y=w1225) -> (x+y=w1227:i32)
                          n948 = Bundle("y"=1775, w1227) -> (w1226:cluster{"y":i32, i32})  [unwired: 1 in]
                          n949 = property class="Bool (严格)"(reference=w1231, "Position"=w1226) -> ()  [unwired: 1 in, 2 out]
                        }
                        n950 = Build Array(w1201, w1200, w1199, w1195, w1198, w1197, w1196) -> (w1202:refnum<vi>[])
                        n951 = control-ref of="控制器支架螺栓2拧紧确认"() -> (w1205:refnum<vi>)
                        n952 = control-ref of="控制器支架螺栓1拧紧确认"() -> (w1206:refnum<vi>)
                        n953 = control-ref of="控制器支架螺栓3拧紧确认"() -> (w1204:refnum<vi>)
                        n954 = control-ref of="控制器支架螺栓4拧紧确认"() -> (w1203:refnum<vi>)
                        n955 = control-ref of="控制器支架涂色标"() -> (w1185:refnum<vi>)
                        n956 = for {
                          tunnel: w1202 -> [w1215] mode=indexing
                          i -> [w1214]
                          n957 = Multiply(x=60, y=w1214) -> (x*y=w1212:i32)
                          n958 = Add(x=w1212, y=340) -> (x+y=w1209:i32)
                          n959 = Bundle("y"=2115, w1209) -> (w1208:cluster{"y":i32, i32})  [unwired: 1 in]
                          n960 = property class="Bool (严格)"(reference=w1215, "Position"=w1208) -> ()  [unwired: 1 in, 2 out]
                        }
                        n961 = Build Array(w1206, w1205, w1204, w1203, w1185) -> (w1207:refnum<vi>[])
                        n962 = for {
                          tunnel: w1207 -> [w1223] mode=indexing
                          i -> [w1222]
                          n963 = Multiply(x=60, y=w1222) -> (x*y=w1220:i32)
                          n964 = Add(x=w1220, y=345) -> (x+y=w1217:i32)
                          n965 = Bundle("y"=1445, w1217) -> (w1216:cluster{"y":i32, i32})  [unwired: 1 in]
                          n966 = property class="Bool (严格)"(reference=w1223, "Position"=w1216) -> ()  [unwired: 1 in, 2 out]
                        }
                      }
                      frame "R128" {
                        # "1345"
                        n967 = control-ref of="请取锁紧块"() -> (w1247:refnum<vi>)
                        n968 = control-ref of="请安装锁紧螺母"() -> (w1246:refnum<vi>)
                        n969 = control-ref of="请取降噪块2"() -> (w1248:refnum<vi>)
                        n970 = control-ref of="?"() -> (w1250:refnum<vi>)
                        n971 = control-ref of="?"() -> (w1249:refnum<vi>)
                        n972 = control-ref of="安装弹性垫圈弹簧并按启动拍照"() -> (w1241:refnum<vi>)
                        n973 = control-ref of="电机安装螺栓1扭矩确认"() -> (w1240:refnum<vi>)
                        n974 = control-ref of="电机安装螺栓2扭矩确认"() -> (w1239:refnum<vi>)
                        n975 = control-ref of="涂色标"() -> (w1237:refnum<vi>)
                        n976 = control-ref of="安装扎带并取走工件"() -> (w1236:refnum<vi>)
                        n977 = control-ref of="按启动按钮拍照确认"() -> (w1238:refnum<vi>)
                        n978 = Build Array(w1250, w1249, w1248, w1247, w1246) -> (w1253:refnum<vi>[])
                        n979 = control-ref of="控制器支架螺栓2拧紧确认"() -> (w1244:refnum<vi>)
                        n980 = control-ref of="控制器支架螺栓1拧紧确认"() -> (w1245:refnum<vi>)
                        n981 = control-ref of="控制器支架螺栓3拧紧确认"() -> (w1243:refnum<vi>)
                        n982 = control-ref of="控制器支架螺栓5拧紧确认"() -> ()  [unwired: 1 out]
                        n983 = control-ref of="控制器支架涂色标"() -> (w1235:refnum<vi>)
                        n984 = control-ref of="控制器支架螺栓4拧紧确认"() -> (w1242:refnum<vi>)
                        n985 = for {
                          tunnel: w1253 -> [w1285] mode=indexing
                          i -> [w1284]
                          n986 = Multiply(x=60, y=w1284) -> (x*y=w1279:i32)
                          n987 = Add(x=438 ("y"), y=w1279) -> (x+y=w1281:i32)
                          n988 = Bundle("y"=-1495, w1281) -> (w1280:cluster{"y":i32, i32})  [unwired: 1 in]
                          n989 = property class="Bool (严格)"(reference=w1285, "Position"=w1280) -> ()  [unwired: 1 in, 2 out]
                        }
                        n990 = Build Array(w1241, w1240, w1239, w1238, w1237, w1236) -> (w1251:refnum<vi>[])
                        n991 = for {
                          tunnel: w1251 -> [w1269] mode=indexing
                          i -> [w1268]
                          n992 = Multiply(x=60, y=w1268) -> (x*y=w1266:i32)
                          n993 = Add(x=w1266, y=438) -> (x+y=w1263:i32)
                          n994 = Bundle("y"=-1145, w1263) -> (w1262:cluster{"y":i32, i32})  [unwired: 1 in]
                          n995 = property class="Bool (严格)"(reference=w1269, "Position"=w1262) -> ()  [unwired: 1 in, 2 out]
                        }
                        n996 = control-ref of="请安装推力滚针轴承"() -> (w1234:refnum<vi>)
                        n997 = Build Array(w1245, w1244, w1243, w1242, w1235) -> (w1252:refnum<vi>[])
                        n998 = control-ref of="请安装挡片"() -> (w1232:refnum<vi>)
                        n999 = for {
                          tunnel: w1252 -> [w1277] mode=indexing
                          i -> [w1276]
                          n1000 = Multiply(x=60, y=w1276) -> (x*y=w1274:i32)
                          n1001 = Add(x=w1274, y=438) -> (x+y=w1271:i32)
                          n1002 = Bundle("y"=-1820, w1271) -> (w1270:cluster{"y":i32, i32})  [unwired: 1 in]
                          n1003 = property class="Bool (严格)"(reference=w1277, "Position"=w1270) -> ()  [unwired: 1 in, 2 out]
                        }
                        n1004 = Build Array(w1234, w1232) -> (w1233:refnum<vi>[])
                        n1005 = for {
                          tunnel: w1233 -> [w1261] mode=indexing
                          i -> [w1260]
                          n1006 = Multiply(x=60, y=w1260) -> (x*y=w1258:i32)
                          n1007 = Add(x=w1258, y=438) -> (x+y=w1255:i32)
                          n1008 = Bundle("y"=-100, w1255) -> (w1254:cluster{"y":i32, i32})  [unwired: 1 in]
                          n1009 = property class="Bool (严格)"(reference=w1261, "Position"=w1254) -> ()  [unwired: 1 in, 2 out]
                        }
                      }
                      frame "R092B" {
                        # "1345"
                        n1010 = control-ref of="请安装推力滚针轴承"() -> (w1286:refnum<vi>)
                        n1011 = control-ref of="请安装锁紧螺母"() -> (w1298:refnum<vi>)
                        n1012 = control-ref of="请取锁紧块"() -> (w1299:refnum<vi>)
                        n1013 = control-ref of="请取降噪块2"() -> (w1300:refnum<vi>)
                        n1014 = control-ref of="?"() -> (w1302:refnum<vi>)
                        n1015 = control-ref of="?"() -> (w1301:refnum<vi>)
                        n1016 = control-ref of="安装弹性垫圈弹簧并按启动拍照"() -> (w1293:refnum<vi>)
                        n1017 = control-ref of="电机安装螺栓1扭矩确认"() -> (w1292:refnum<vi>)
                        n1018 = control-ref of="电机安装螺栓2扭矩确认"() -> (w1291:refnum<vi>)
                        n1019 = control-ref of="涂色标"() -> (w1289:refnum<vi>)
                        n1020 = control-ref of="安装扎带并取走工件"() -> (w1288:refnum<vi>)
                        n1021 = control-ref of="按启动按钮拍照确认"() -> (w1290:refnum<vi>)
                        n1022 = Build Array(w1302, w1301, w1300, w1299, w1286, w1298) -> (w1305:refnum<vi>[])
                        n1023 = control-ref of="控制器支架螺栓2拧紧确认"() -> (w1296:refnum<vi>)
                        n1024 = control-ref of="控制器支架螺栓1拧紧确认"() -> (w1297:refnum<vi>)
                        n1025 = control-ref of="控制器支架螺栓3拧紧确认"() -> (w1295:refnum<vi>)
                        n1026 = control-ref of="控制器支架涂色标"() -> (w1287:refnum<vi>)
                        n1027 = control-ref of="控制器支架螺栓4拧紧确认"() -> (w1294:refnum<vi>)
                        n1028 = for {
                          tunnel: w1305 -> [w1329] mode=indexing
                          i -> [w1328]
                          n1029 = Multiply(x=60, y=w1328) -> (x*y=w1323:i32)
                          n1030 = Add(x=438 ("y"), y=w1323) -> (x+y=w1325:i32)
                          n1031 = Bundle("y"=-1495, w1325) -> (w1324:cluster{"y":i32, i32})  [unwired: 1 in]
                          n1032 = property class="Bool (严格)"(reference=w1329, "Position"=w1324) -> ()  [unwired: 1 in, 2 out]
                        }
                        n1033 = Build Array(w1293, w1292, w1291, w1290, w1289, w1288) -> (w1303:refnum<vi>[])
                        n1034 = for {
                          tunnel: w1303 -> [w1313] mode=indexing
                          i -> [w1312]
                          n1035 = Multiply(x=60, y=w1312) -> (x*y=w1310:i32)
                          n1036 = Add(x=w1310, y=438) -> (x+y=w1307:i32)
                          n1037 = Bundle("y"=-1145, w1307) -> (w1306:cluster{"y":i32, i32})  [unwired: 1 in]
                          n1038 = property class="Bool (严格)"(reference=w1313, "Position"=w1306) -> ()  [unwired: 1 in, 2 out]
                        }
                        n1039 = Build Array(w1297, w1296, w1295, w1294, w1287) -> (w1304:refnum<vi>[])
                        n1040 = control-ref of="控制器支架螺栓5拧紧确认"() -> ()  [unwired: 1 out]
                        n1041 = for {
                          tunnel: w1304 -> [w1321] mode=indexing
                          i -> [w1320]
                          n1042 = Multiply(x=60, y=w1320) -> (x*y=w1318:i32)
                          n1043 = Add(x=w1318, y=438) -> (x+y=w1315:i32)
                          n1044 = Bundle("y"=-1820, w1315) -> (w1314:cluster{"y":i32, i32})  [unwired: 1 in]
                          n1045 = property class="Bool (严格)"(reference=w1321, "Position"=w1314) -> ()  [unwired: 1 in, 2 out]
                        }
                      }
                      frame "R563X" {
                        # "1345"
                        n1046 = control-ref of="请取锁紧块"() -> (w1349:refnum<vi>)
                        n1047 = control-ref of="请安装锁紧螺母"() -> (w1348:refnum<vi>)
                        n1048 = control-ref of="请取降噪块2"() -> (w1350:refnum<vi>)
                        n1049 = control-ref of="?"() -> (w1352:refnum<vi>)
                        n1050 = control-ref of="?"() -> (w1351:refnum<vi>)
                        n1051 = control-ref of="安装弹性垫圈弹簧并按启动拍照"() -> (w1344:refnum<vi>)
                        n1052 = control-ref of="电机安装螺栓1扭矩确认"() -> (w1343:refnum<vi>)
                        n1053 = control-ref of="电机安装螺栓2扭矩确认"() -> (w1342:refnum<vi>)
                        n1054 = control-ref of="涂色标"() -> (w1340:refnum<vi>)
                        n1055 = control-ref of="安装扎带并取走工件"() -> (w1339:refnum<vi>)
                        n1056 = control-ref of="按启动按钮拍照确认"() -> (w1341:refnum<vi>)
                        n1057 = control-ref of="控制器支架螺栓2拧紧确认"() -> (w1346:refnum<vi>)
                        n1058 = control-ref of="控制器支架螺栓1拧紧确认"() -> (w1347:refnum<vi>)
                        n1059 = control-ref of="控制器支架螺栓3拧紧确认"() -> (w1345:refnum<vi>)
                        n1060 = control-ref of="控制器支架涂色标"() -> (w1338:refnum<vi>)
                        n1061 = Build Array(w1352, w1351, w1350, w1349, w1348) -> (w1355:refnum<vi>[])
                        n1062 = control-ref of="控制器支架螺栓5拧紧确认"() -> (w1333:refnum<vi>)
                        n1063 = control-ref of="控制器支架螺栓4拧紧确认"() -> (w1332:refnum<vi>)
                        n1064 = control-ref of="请安装弹簧"() -> (w1331:refnum<vi>)
                        n1065 = for {
                          tunnel: w1355 -> [w1387] mode=indexing
                          i -> [w1386]
                          n1066 = Multiply(x=60, y=w1386) -> (x*y=w1381:i32)
                          n1067 = Add(x=438 ("y"), y=w1381) -> (x+y=w1383:i32)
                          n1068 = Bundle("y"=-1495, w1383) -> (w1382:cluster{"y":i32, i32})  [unwired: 1 in]
                          n1069 = property class="Bool (严格)"(reference=w1387, "Position"=w1382) -> ()  [unwired: 1 in, 2 out]
                        }
                        n1070 = Build Array(w1344, w1343, w1342, w1341, w1340, w1339) -> (w1353:refnum<vi>[])
                        n1071 = control-ref of="安装支架扎带安装"() -> (w1334:refnum<vi>)
                        n1072 = control-ref of="请拍照确认"() -> (w1335:refnum<vi>)
                        n1073 = control-ref of="控制器支架安装线卡扎带"() -> ()  [unwired: 1 out]
                        n1074 = control-ref of="控制器支架螺栓5拧紧确认"() -> (w1336:refnum<vi>)
                        n1075 = control-ref of="控制器支架螺栓4拧紧确认"() -> (w1337:refnum<vi>)
                        n1076 = for {
                          tunnel: w1353 -> [w1371] mode=indexing
                          i -> [w1370]
                          n1077 = Multiply(x=60, y=w1370) -> (x*y=w1368:i32)
                          n1078 = Add(x=w1368, y=438) -> (x+y=w1365:i32)
                          n1079 = Bundle("y"=-1145, w1365) -> (w1364:cluster{"y":i32, i32})  [unwired: 1 in]
                          n1080 = property class="Bool (严格)"(reference=w1371, "Position"=w1364) -> ()  [unwired: 1 in, 2 out]
                        }
                        n1081 = Build Array(w1347, w1346, w1345, w1338) -> (w1354:refnum<vi>[])
                        n1082 = Build Array(w1337, w1336, w1335, w1334, w1333, w1332, w1331) -> (w1330:refnum<vi>[])
                        n1083 = for {
                          tunnel: w1354 -> [w1379] mode=indexing
                          i -> [w1378]
                          n1084 = Multiply(x=60, y=w1378) -> (x*y=w1376:i32)
                          n1085 = Add(x=w1376, y=438) -> (x+y=w1373:i32)
                          n1086 = Bundle("y"=-1820, w1373) -> (w1372:cluster{"y":i32, i32})  [unwired: 1 in]
                          n1087 = property class="Bool (严格)"(reference=w1379, "Position"=w1372) -> ()  [unwired: 1 in, 2 out]
                        }
                        n1088 = for {
                          tunnel: w1330 -> [w1363] mode=indexing
                          i -> [w1362]
                          n1089 = Multiply(x=60, y=w1362) -> (x*y=w1360:i32)
                          n1090 = Add(x=w1360, y=438) -> (x+y=w1357:i32)
                          n1091 = Bundle("y"=-100, w1357) -> (w1356:cluster{"y":i32, i32})  [unwired: 1 in]
                          n1092 = property class="Bool (严格)"(reference=w1363, "Position"=w1356) -> ()  [unwired: 1 in, 2 out]
                        }
                      }
                    }
                  }
                  frame Enabled {
                  }
                }
              }
            }
          }
          event "更换产品": Value Change {
            n1093 = event-data() -> ()  [unwired: 1 in, 6 out]
            n1094 = global read "Global.vi" "产品型号"() -> (w1388:string)
            n1095 = case shown="\"R563X\", 默认" w1388 {
              frame "R563X", Default {
                n1096 = control-ref of="?"() -> (w1427:refnum<vi>)
                n1097 = control-ref of="?"() -> (w1429:refnum<vi>)
                n1098 = property class="Bool (严格)"(reference=w1429, "Caption.Text"="请取衬套2" ("标题.文本")) -> ()  [unwired: 1 in, 2 out]
                n1099 = property class="Bool (严格)"(reference=w1427, "Caption.Text"="请取衬套1" ("标题.文本")) -> ()  [unwired: 1 in, 2 out]
              }
              frame "R567X" {
                n1100 = control-ref of="?"() -> (w1431:refnum<vi>)
                n1101 = control-ref of="?"() -> (w1433:refnum<vi>)
                n1102 = property class="Bool (严格)"(reference=w1431, "Caption.Text"="请取降噪垫片2" ("标题.文本")) -> ()  [unwired: 1 in, 2 out]
                n1103 = property class="Bool (严格)"(reference=w1433, "Caption.Text"="请取降噪垫片1" ("标题.文本")) -> ()  [unwired: 1 in, 2 out]
              }
            }
            n1104 = control-ref of="控制器支架安装线卡扎带"() -> (w1419:refnum<vi>)
            n1105 = control-ref of="控制器支架螺栓5拧紧确认"() -> (w1421:refnum<vi>)
            n1106 = control-ref of="控制器支架涂色标"() -> (w1420:refnum<vi>)
            n1107 = control-ref of="控制器支架螺栓3拧紧确认"() -> (w1423:refnum<vi>)
            n1108 = control-ref of="控制器支架螺栓4拧紧确认"() -> (w1422:refnum<vi>)
            n1109 = control-ref of="控制器支架螺栓2拧紧确认"() -> (w1424:refnum<vi>)
            n1110 = control-ref of="控制器支架螺栓1拧紧确认"() -> (w1425:refnum<vi>)
            n1111 = control-ref of="请安装挡片"() -> (w1409:refnum<vi>)
            n1112 = global read "Global.vi" "控制器支架"() -> (w1416:bool[])
            n1113 = control-ref of="请安装弹簧"() -> (w1408:refnum<vi>)
            n1114 = control-ref of="请取锁紧块"() -> (w1411:refnum<vi>)
            n1115 = control-ref of="请安装推力滚针轴承"() -> (w1410:refnum<vi>)
            n1116 = control-ref of="请安装锁紧螺母"() -> (w1407:refnum<vi>)
            n1117 = control-ref of="请拍照确认"() -> (w1406:refnum<vi>)
            n1118 = control-ref of="?"() -> (w1414:refnum<vi>)
            n1119 = control-ref of="请取降噪块2"() -> (w1412:refnum<vi>)
            n1120 = control-ref of="请取降噪块1"() -> (w1413:refnum<vi>)
            n1121 = control-ref of="?"() -> (w1415:refnum<vi>)
            n1122 = Build Array(w1425, w1424, w1423, w1422, w1421, w1420, w1419) -> (w1391:refnum<vi>[])
            n1123 = for "For循环" {
              tunnel: w1416 -> [w1467] mode=indexing
              tunnel: w1391 -> [w1466] mode=indexing
              shift-right: [w1464] -> _
              shift-left: 360 -> [w1465]
              tunnel: w1391 -> [w1463]
              i -> [w1462]
              n1124 = case shown="假" w1467 {
                tunnel: w1466 -> [w1469 w1471]
                tunnel: w1465 -> [w1470 w1476]
                tunnel: [w1470 w1473] -> w1464
                tunnel: w1463 -> [_ _]
                tunnel: w1462 -> [_ _]
                frame False {
                  n1125 = property class="Bool (严格)"(reference=w1469, "Top"=-100 ("位置:置顶")) -> ()  [unwired: 1 in, 2 out]
                }
                frame True {
                  n1126 = Add(x=w1476, y=50) -> (x+y=w1473:i32)
                  n1127 = Bundle(-1850, w1473) -> (w1474:cluster{i32, i32})  [unwired: 1 in]
                  n1128 = property class="Bool (严格)"(reference=w1471, "Position"=w1474) -> ()  [unwired: 1 in, 2 out]
                }
              }
            }
            n1129 = global read "Global.vi" "手柄安装步骤"() -> (w1405:bool[])
            n1130 = Build Array(w1415, w1414, w1413, w1412, w1411, w1410, w1409, w1407, w1408, w1406) -> (w1404:refnum<vi>[])
            n1131 = for "For循环" {
              tunnel: w1405 -> [w1452] mode=indexing
              tunnel: w1404 -> [w1451] mode=indexing
              shift-right: [w1449] -> _
              shift-left: 360 -> [w1450]
              tunnel: w1404 -> [w1448]
              n1132 = case shown="真" w1452 {
                tunnel: w1451 -> [w1454 w1456]
                tunnel: w1450 -> [w1455 w1461]
                tunnel: [w1455 w1458] -> w1449
                tunnel: w1448 -> [_ _]
                frame False {
                  n1133 = property class="Bool (严格)"(reference=w1454, "Top"=-100 ("位置:置顶")) -> ()  [unwired: 1 in, 2 out]
                }
                frame True {
                  n1134 = Add(x=w1461, y=70) -> (x+y=w1458:i32)
                  n1135 = Bundle(-1510, w1458) -> (w1459:cluster{i32, i32})  [unwired: 1 in]
                  n1136 = property class="Bool (严格)"(reference=w1456, "Position"=w1459) -> ()  [unwired: 1 in, 2 out]
                }
              }
            }
            n1137 = control-ref of="电机安装螺栓1扭矩确认"() -> (w1401:refnum<vi>)
            n1138 = control-ref of="安装弹性垫圈弹簧并按启动拍照"() -> (w1402:refnum<vi>)
            n1139 = control-ref of="请拾取O型圈"() -> (w1390:refnum<vi>)
            n1140 = control-ref of="请拾取弹簧"() -> (w1389:refnum<vi>)
            n1141 = control-ref of="安装扎带并取走工件"() -> (w1395:refnum<vi>)
            n1142 = control-ref of="电机安装螺栓3扭矩确认"() -> (w1399:refnum<vi>)
            n1143 = control-ref of="电机安装螺栓2扭矩确认"() -> (w1400:refnum<vi>)
            n1144 = control-ref of="按启动按钮拍照确认"() -> (w1398:refnum<vi>)
            n1145 = control-ref of="安装支架扎带安装"() -> (w1396:refnum<vi>)
            n1146 = control-ref of="涂色标"() -> (w1397:refnum<vi>)
            n1147 = global read "Global.vi" "电机安装"() -> (w1393:bool[])
            n1148 = Build Array(w1389, w1390, w1402, w1401, w1400, w1399, w1398, w1397, w1396, w1395) -> (w1394:refnum<vi>[])
            n1149 = for "For循环" {
              tunnel: w1393 -> [w1438] mode=indexing
              tunnel: w1394 -> [w1437] mode=indexing
              shift-right: [w1435] -> _
              shift-left: 360 -> [w1436]
              tunnel: w1394 -> [w1434]
              n1150 = case shown="真" w1438 {
                tunnel: w1437 -> [w1440 w1442]
                tunnel: w1436 -> [w1441 w1447]
                tunnel: [w1441 w1444] -> w1435
                tunnel: w1434 -> [_ _]
                frame False {
                  n1151 = property class="Bool (严格)"(reference=w1440, "Top"=-100 ("位置:置顶")) -> ()  [unwired: 1 in, 2 out]
                }
                frame True {
                  n1152 = Add(x=w1447, y=50) -> (x+y=w1444:i32)
                  n1153 = Bundle(-1193, w1444) -> (w1445:cluster{i32, i32})  [unwired: 1 in]
                  n1154 = property class="Bool (严格)"(reference=w1442, "Position"=w1445) -> ()  [unwired: 1 in, 2 out]
                }
              }
            }
            "产品型号" <- w1417
          }
          event Panel Close {
            n1155 = event-data() -> ()  [unwired: 1 in, 4 out]
            n1156 = global write "Global.vi" "程序关闭"(TRUE ("程序关闭")) -> ()
          }
        }
        n1157 = case shown="真" w1110 {
          tunnel: w1109 -> [_ w1112]
          frame False {
          }
          frame True {
            n1158 = property on="更换布局" class="Str"("Val(Sgnl)"=w1112) -> ()  [unwired: 2 in, 2 out]
          }
        }
        n1159 = control-ref of="更换产品"() -> (w1107:refnum<vi>)
        n1160 = global write "Global.vi" "更换产品"(w1107) -> ()
        n1161 = global read "Global.vi" "程序关闭"() -> (w1108:bool)
      }
    }
  }
